vi "运维调试_质控单元.vi"() -> ()   [LabVIEW 2016, in "质控单元.lvlib"]
uses:
  <vilib>/Utility/miscctls.llb/LVPointTypeDef.ctl
  <vilib>/Utility/config.llb/Read Key (I32).vi
  <vilib>/Utility/config.llb/Read Key (Boolean).vi
  <vilib>/Utility/config.llb/Read Key (U32).vi
  <vilib>/Utility/config.llb/Write Key (I32).vi
  <vilib>/Utility/config.llb/Write Key (Boolean).vi
  <vilib>/Utility/config.llb/NI_LVConfig.lvlib
panel:
  in  "标样核查量程选择":enum32{"H", "L", "AUTO"}(ring)=enum."AUTO"
  in  "零点核查量程选择":enum32{"H", "L", "AUTO"}(ring)=enum."AUTO"
  in  "跨度量程选择":enum32{"H", "L", "AUTO"}(ring)=enum."AUTO"
  in  "定时启动":bool
  out "串口/TCP":string
  out "CODCr状态簇":T1
  out "CODMn状态簇":T1
  out "总氮状态簇":T1
  out "总磷状态簇":T1
  out "氨氮状态簇":T1
  out "总氮柱塞泵故障报警":bool
  out "CODCr柱塞泵故障报警":bool
  out "CODMn柱塞泵故障报警":bool
  out "总磷柱塞泵故障报警":bool
  out "氨氮柱塞泵故障报警":bool
  out "总氮传感器故障报警":bool
  out "总氮传感器状态":bool
  out "总氮流程中断报警":bool
  out "总磷通讯":bool
  out "CODCr质控流程中":bool
  out "CODMn质控流程中":bool
  out "总氮质控流程中":bool caption="总磷质控流程中"
  out "总磷质控流程中":bool caption="总氮质控流程中"
  out "氨氮质控流程中":bool
  out "CODCr通讯":bool
  out "CODMn通讯":bool
  out "总氮通讯":bool
  out "氨氮通讯":bool
  out "CODCr传感器状态":bool
  out "CODCr传感器故障报警":bool
  out "CODMn传感器故障报警":bool
  out "总磷传感器故障报警":bool
  out "氨氮传感器故障报警":bool
  out "CODMn传感器状态":bool
  out "总磷传感器状态":bool
  out "氨氮传感器状态":bool
  out "CODCr流程中断报警":bool
  out "总磷流程中断报警":bool
  out "CODMn流程中断报警":bool
  out "氨氮流程中断报警":bool
  in  "总氮模块选择":bool
  in  "释放串口":bool
  in  "打开串口":bool
  in  "柱塞泵调试":bool
  in  "手动调试":bool
  in  "报警清除":bool
  in  "查看":bool
  in  "停止测量":bool
  in  "加标回收":bool
  in  "平行样测试":bool
  in  "CODCr量程选择":enum32{"H", "L", "AUTO"}(ring)
  in  "CODCr选择":bool
  out "CODCr加标回收率":dbl caption="加标回收率" format="%.2f"
  out "CODCr加标体积":dbl caption="加标体积" format="%.3f"
  out "CODCr母液浓度":dbl caption="加标母液浓度" format="%.2f"
  out "CODCr加标水杯定容体积":dbl caption="加标水杯定容体积" format="%.2f"
  out "CODCr加标后水样浓度":dbl caption="加标后水样浓度" format="%.2f"
  out "CODCr加标前水样浓度":dbl caption="加标前水样浓度" format="%.2f"
  out "CODCr检出限":dbl caption="检出限" format="%.2f"
  out "CODCr量程":dbl caption="量程" format="%.2f"
  out "CODCr状态":u16(ring) caption="状态" items=["待机", "润洗", "进样", "进样完成", "柱塞泵加标", "等待取液", "排液"]
  out "质控流程中":bool
  in  "CODMn量程选择":enum32{"H", "L", "AUTO"}(ring)
  in  "总磷量程选择":enum32{"H", "L", "AUTO"}(ring)=enum."AUTO"
  in  "总氮量程选择":enum32{"H", "L", "AUTO"}(ring)=enum."AUTO"
  in  "氨氮量程选择":enum32{"H", "L", "AUTO"}(ring)=enum."AUTO"
  in  "CODMn选择":bool
  in  "总磷模块选择":bool
  in  "氨氮模块":bool
  in  "背隙补偿步数 3":i32 min=0 max=2000
  in  "背隙补偿步数 2":i32 min=0 max=2000
  in  "背隙补偿步数":i32 min=0 max=2000
  out "总氮加标回收率":dbl caption="加标回收率" format="%.2f"
  out "总氮加标体积":dbl caption="加标体积" format="%.3f"
  out "总氮母液浓度":dbl caption="加标母液浓度" format="%.3f"
  out "总氮加标水杯定容体积":dbl caption="加标水杯定容体积" format="%.2f"
  out "总氮加标后水样浓度":dbl caption="加标后水样浓度" format="%.3f"
  out "总氮加标前水样浓度":dbl caption="加标前水样浓度" format="%.3f"
  out "总氮检出限":dbl caption="检出限" format="%.3f"
  out "总氮量程":dbl caption="量程" format="%.2f"
  out "总氮状态":u16(ring) caption="状态" items=["待机", "润洗", "进样", "进样完成", "柱塞泵加标", "等待取液", "排液"]
  in  "返回":bool
  out "COD平行样测完标志":bool
  out "氨氮总磷平行样测完标志":bool
  out "COD加标回收率":dbl caption="加标回收率" format="%.2f"
  out "COD加标体积":dbl caption="加标体积" format="%.3f"
  out "COD母液浓度":dbl caption="加标母液浓度" format="%.2f"
  out "COD加标水杯定容体积":dbl caption="加标水杯定容体积" format="%.2f"
  out "COD加标后水样浓度":dbl caption="加标后水样浓度" format="%.2f"
  out "COD加标前水样浓度":dbl caption="加标前水样浓度" format="%.2f"
  out "COD检出限":dbl caption="检出限" format="%.2f"
  out "COD量程":dbl caption="量程" format="%.2f"
  out "CODMn状态":u16(ring) caption="状态" items=["待机", "润洗", "进样", "进样完成", "柱塞泵加标", "等待取液", "排液"]
  out "总磷加标回收率":dbl caption="加标回收率" format="%.2f"
  out "总磷加标体积":dbl caption="加标体积" format="%.3f"
  out "总磷母液浓度":dbl caption="加标母液浓度" format="%.3f"
  out "总磷加标水杯定容体积":dbl caption="加标水杯定容体积" format="%.2f"
  out "总磷加标后水样浓度":dbl caption="加标后水样浓度" format="%.3f"
  out "总磷加标前水样浓度":dbl caption="加标前水样浓度" format="%.3f"
  out "总磷检出限":dbl caption="检出限" format="%.3f"
  out "总磷量程":dbl caption="量程" format="%.2f"
  out "总磷状态":u16(ring) caption="状态" items=["待机", "润洗", "进样", "进样完成", "柱塞泵加标", "等待取液", "排液"]
  out "氨氮加标回收率":dbl caption="加标回收率" format="%.2f"
  out "氨氮加标体积":dbl caption="加标体积" format="%.3f"
  out "氨氮母液浓度":dbl caption="加标母液浓度" format="%.3f"
  out "氨氮加标水杯定容体积":dbl caption="加标水杯定容体积" format="%.2f"
  out "氨氮加标后水样浓度":dbl caption="加标后水样浓度" format="%.3f"
  out "氨氮加标前水样浓度":dbl caption="加标前水样浓度" format="%.3f"
  out "氨氮检出限":dbl caption="检出限" format="%.3f"
  out "氨氮量程":dbl caption="量程" format="%.2f"
  out "氨氮状态":u16(ring) caption="状态" items=["待机", "润洗", "进样", "进样完成", "柱塞泵加标", "等待取液", "排液"]
  # "氨氮质控参数"
  # "状态显示区"
  # "参数配置区"
  # "2000步等于1mL\n100步等于0.05mL\n20步等于0.01mL\n2步等于0.001mL\n（初始默认100步）"
  # "柱塞泵调试区"
  # "CODCr质控参数"
  # "%"
  # "mL"
  # "mg/L"
  # "mL"
  # "mg/L"
  # "mg/L"
  # "mg/L"
  # "mg/L"
  # "总氮质控参数"
  # "%"
  # "mL"
  # "mg/L"
  # "mL"
  # "mg/L"
  # "mg/L"
  # "mg/L"
  # "mg/L"
  # "CODMn质控参数"
  # "%"
  # "mL"
  # "mg/L"
  # "mL"
  # "mg/L"
  # "mg/L"
  # "mg/L"
  # "mg/L"
  # "总磷质控参数"
  # "%"
  # "mL"
  # "mg/L"
  # "mL"
  # "mg/L"
  # "mg/L"
  # "mg/L"
  # "mg/L"
  # "%"
  # "mL"
  # "mg/L"
  # "mL"
  # "mg/L"
  # "mg/L"
  # "mg/L"
  # "mg/L"
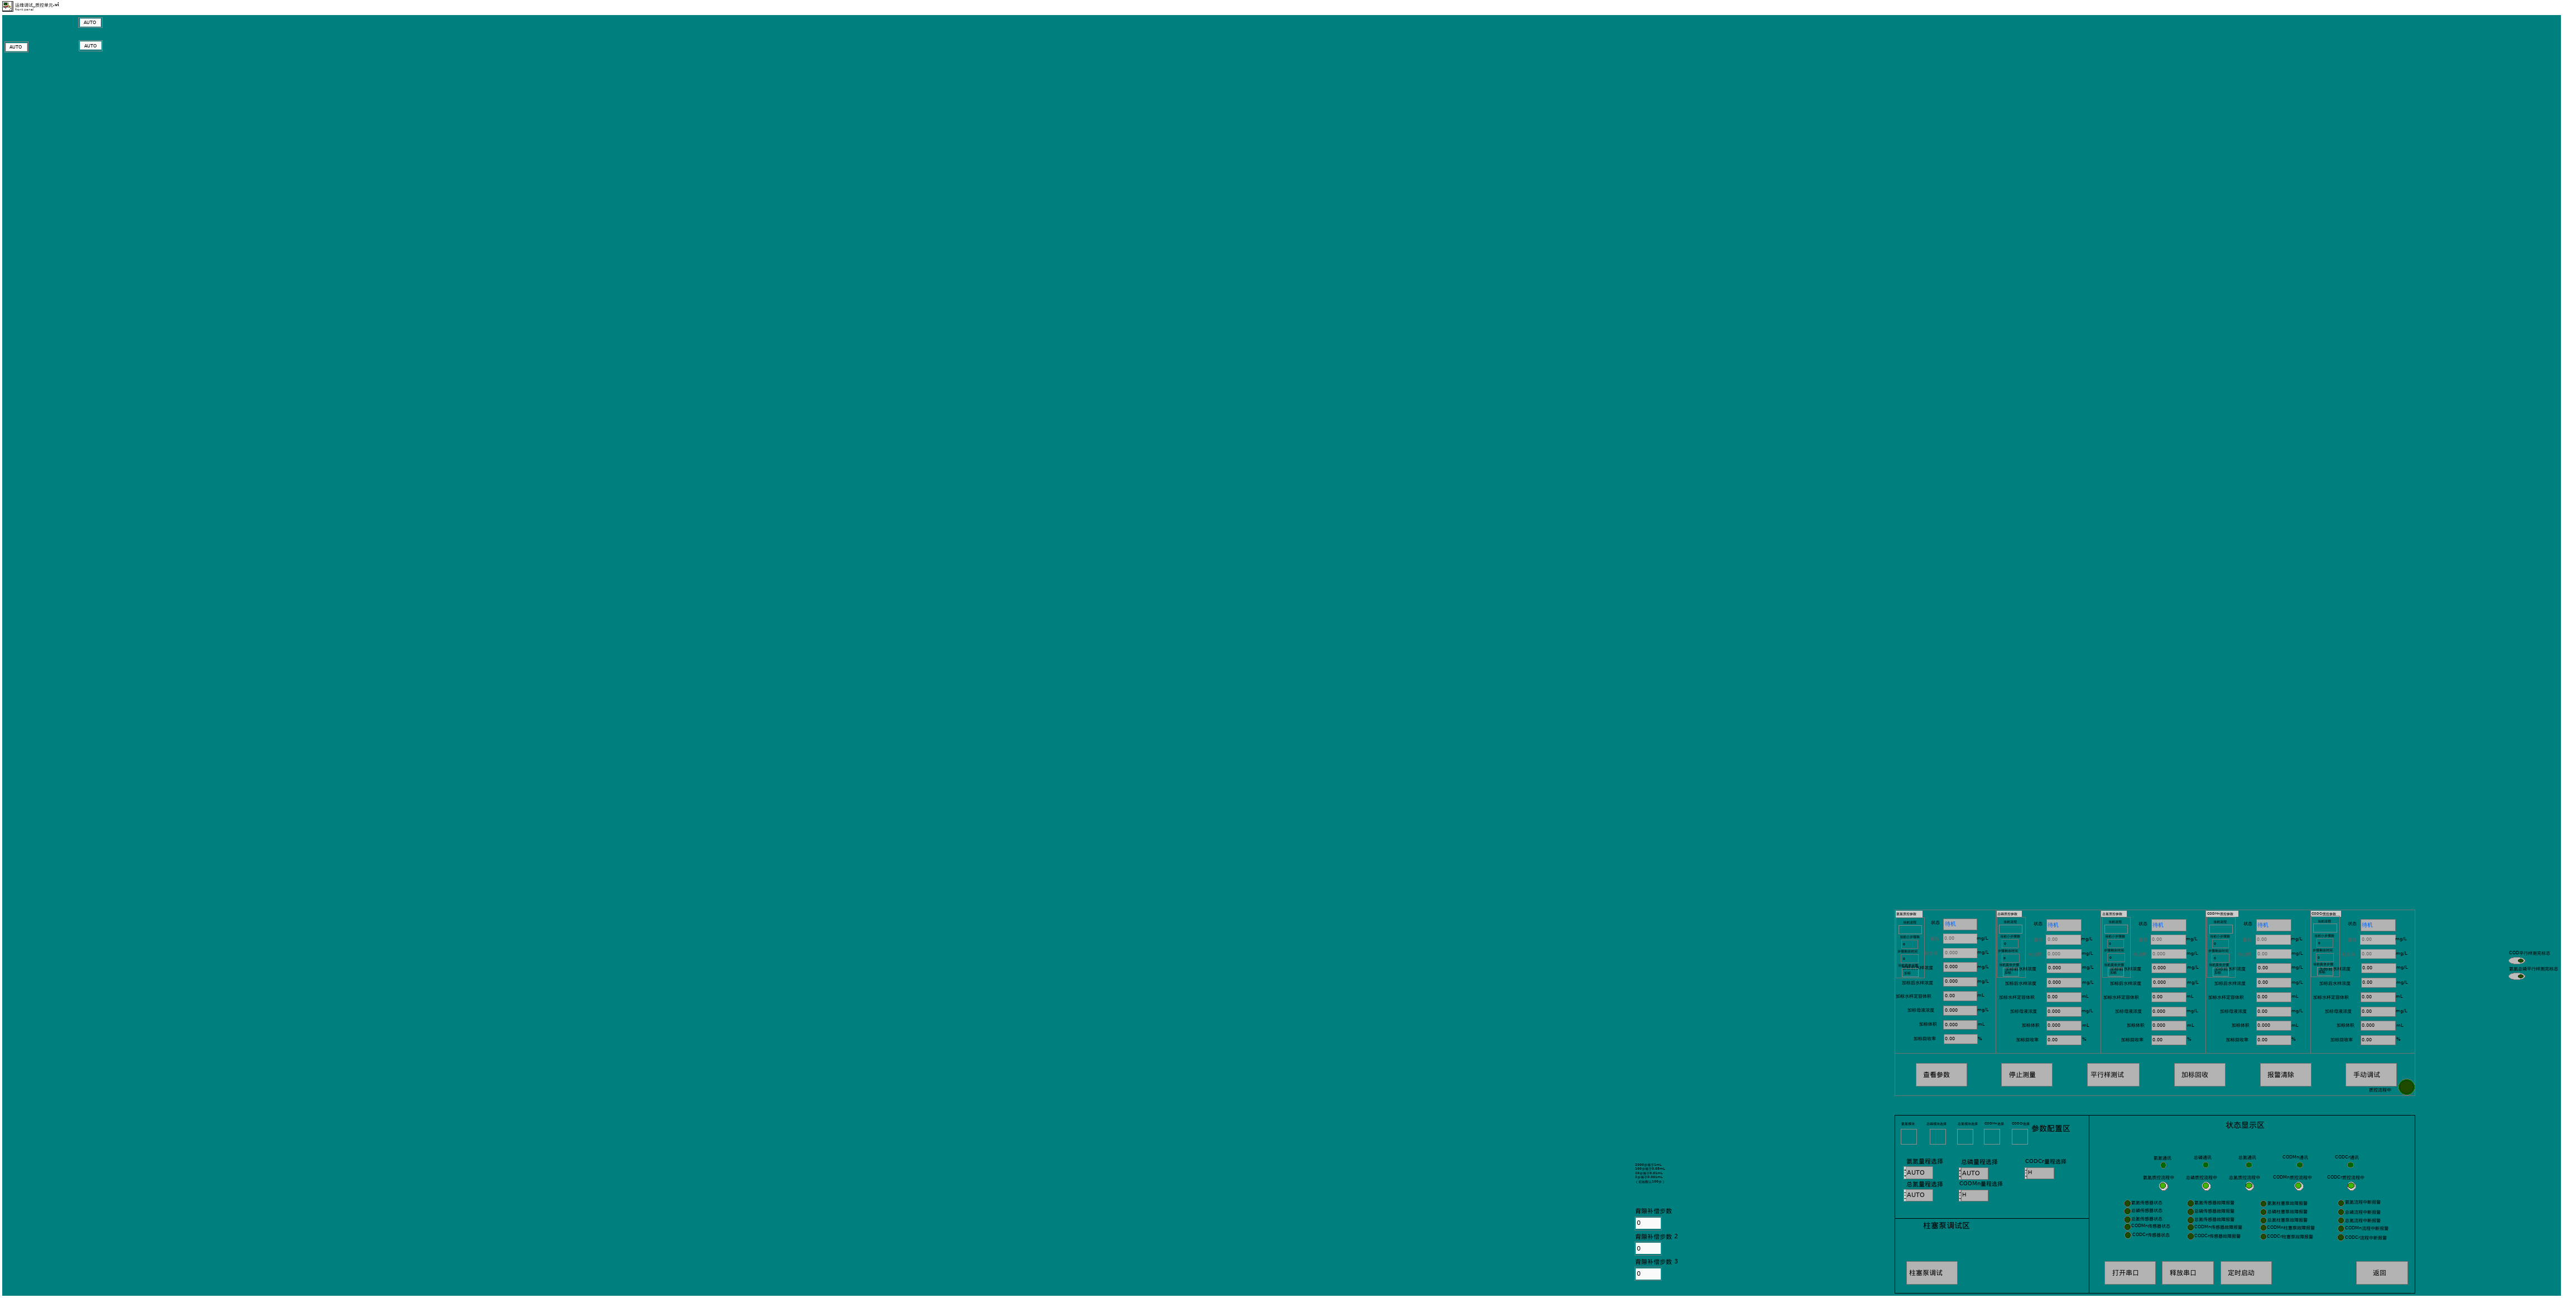
[diagram p1: front panel]
types:
  T1 = cluster{"步骤剩余时间":u16, "当前具体步骤":enum16{"加标", "进样", "排液", "搅拌", "定量"}, " 当前流程":enum16{"", "水样流程", "加标流程", "排液流程"}, "当前小步骤数":i8}
  T2 = typedef "LVPointTypeDef.ctl" = cluster{"Horizontal":i16, "Vertical":i16}
  T3 = typedef "NI_LVConfig.lvlib/Config Data RefNum.ctl" = refnum<k1>
  T4 = cluster{"量程":dbl, "检出限":dbl, "加标前水样浓度":dbl, "加标后水样浓度":dbl, "加标水杯定容体积":dbl, "加标母液浓度":dbl, "加标体积":dbl, "加标回收率":dbl}
  T5 = enum8{"Enabled", "Disabled", "Disabled and Grayed Out"}
  T6 = cluster{"周期设置类型":enum16{"定点启动", "间隔启动"}, "定时功能启用":bool, "定时间隔":dbl, "24H周期设置":bool[], "模块选择":cluster{"氨氮":bool, "总磷":bool, "总氮":bool, "CODMn":bool, "CODCr":bool}}
  T7 = typedef "LVDateTimeRec.ctl" = cluster{"秒数的小数部分":dbl, "秒":i32, "分":i32, "时":i32, "日":i32, "月":i32, "年":i32, "天数（周）":i32, "天数（年）":i32, "DST":i32}
  T8 = cluster{"氨氮":bool, "总磷":bool, "总氮":bool, "CODMn":bool, "CODCr":bool}
  T9 = cluster{"是否启用仪器":bool, "CODMn":cluster{"启动测量模式":cluster{"测量模式":enum16{"水样测量", "标样核查", "加标回收", "平行样", "校零", "校标"}}, "确定按钮":bool}, "启动模块":cluster{"氨氮":bool, "总磷":bool, "总氮":bool, "CODMn":bool, "CODCr":bool}, "常规启动":bool, "直接启动":bool}
  T10 = cluster{"参数启用":cluster{"CODMn":bool, "总磷":bool, "总氮":bool, "氨氮":bool, "CODcr":bool}, "采配水是否启动":bool}
  T11 = cluster{"命令":string, cluster{"starting address":u16, "holding register value":u16}}
  T12 = enum32{"Bad", "Idle", "Run top level", "Running"}
  T13 = cluster{"CODMn":bool, "总磷":bool, "总氮":bool, "氨氮":bool, "CODCr":bool}
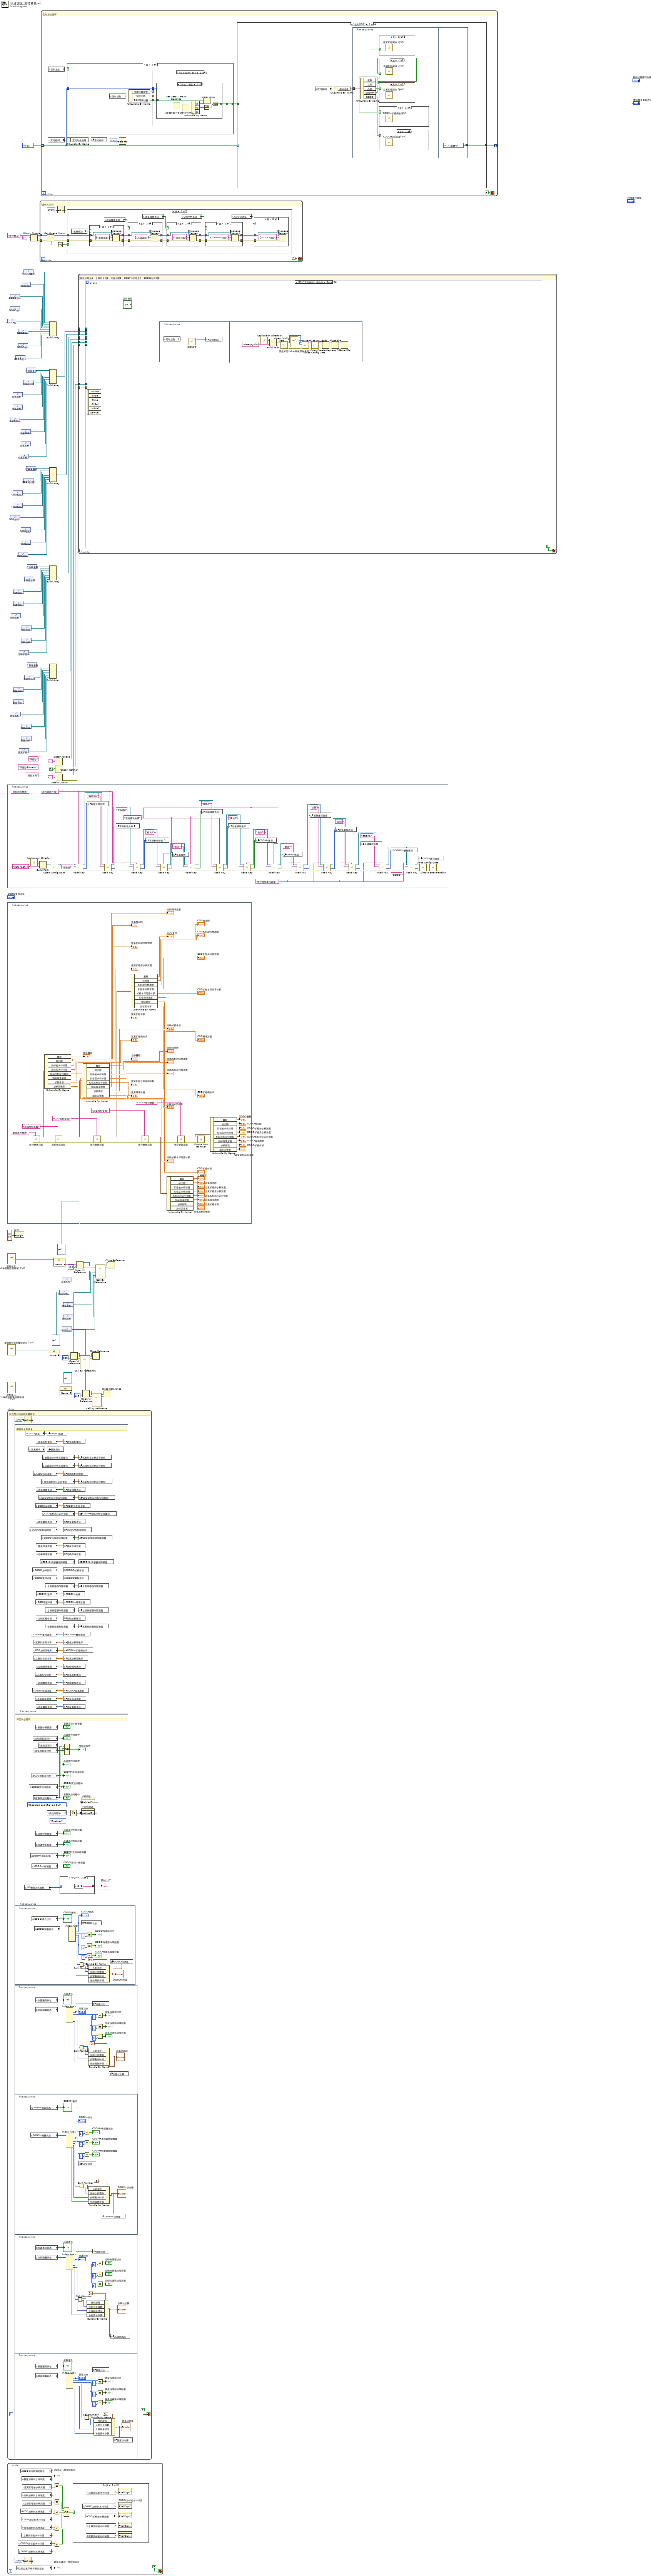
[diagram p0: block diagram]
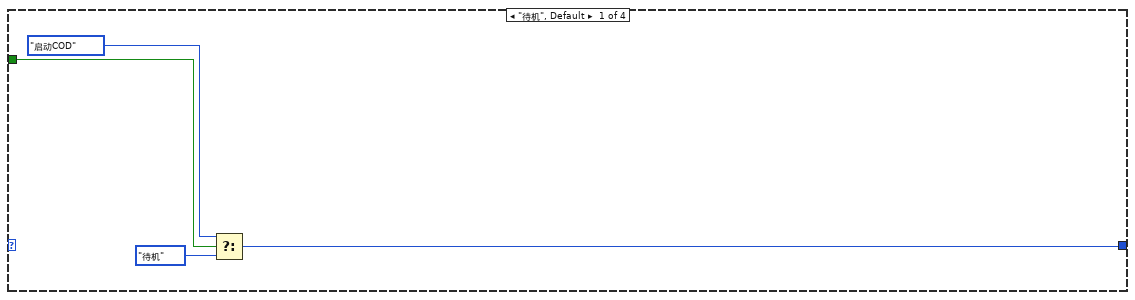
[diagram p2: hidden frame]
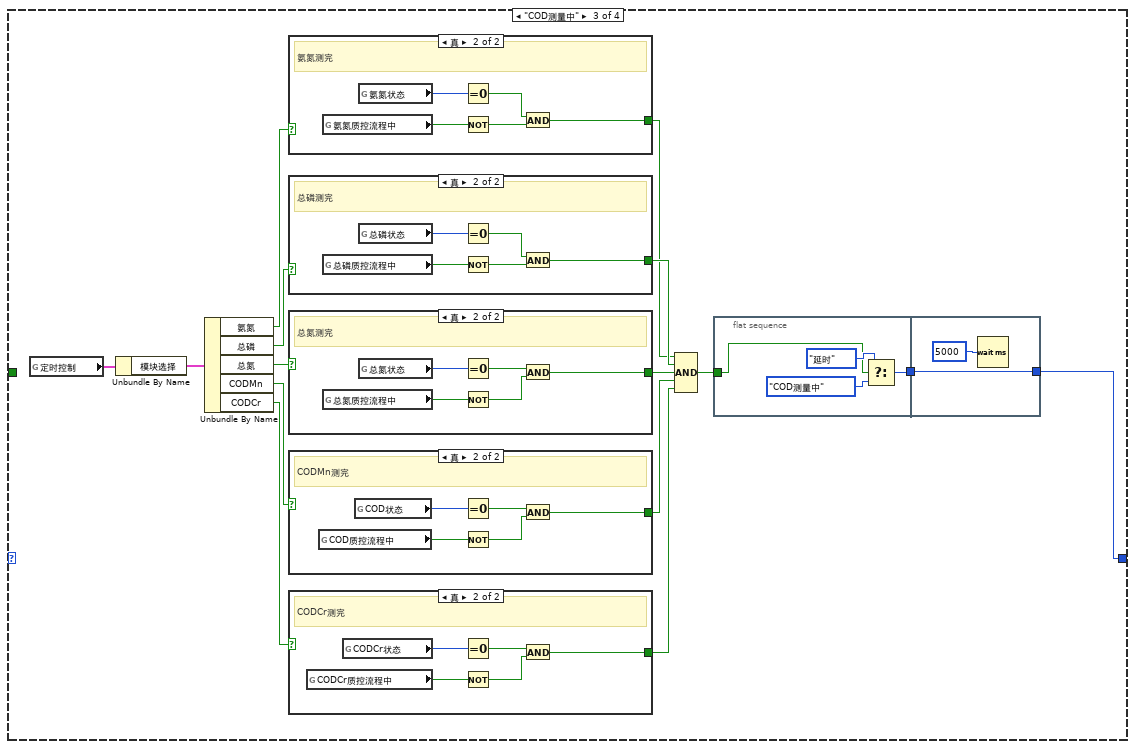
[diagram p8: hidden frame]
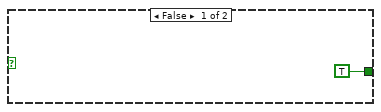
[diagram p9: hidden frame]
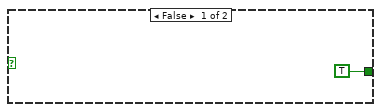
[diagram p10: hidden frame]
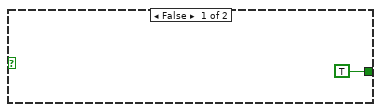
[diagram p11: hidden frame]
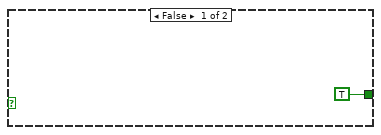
[diagram p12: hidden frame]
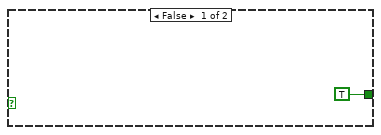
[diagram p13: hidden frame]
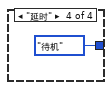
[diagram p14: hidden frame]
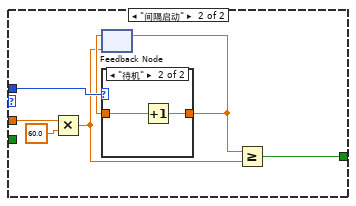
[diagram p17: hidden frame]
diagram:
  n1 = control-ref of="CODCr加标水杯定容体积"() -> (w43:refnum<vi>)
  n2 = flat-sequence {
    frame #0 {
      w111 = "质控模块量程选择" ("section")
      w92 = "质控模块选择" ("section")
      (unwired) "质控线性参数" ("section")
      w145 = "质控背隙补偿" ("section")
      n3 = call <vilib>:"Application Directory.vi"() -> ("Application Directory"=w151:path)
      n4 = Build Path(base path=w151, name or relative path="data\\Set.ini" ("名称或相对路径")) -> (appended path=w149:path)
      n5 = call <vilib>:"Open Config Data.vi"("configuration file path"=w149) -> ("error out"=w147:errorcluster, "refnum"=w148:T3)  [unwired: 8 in, 1 out]
      n6 = call-poly <vilib>:"Read Key.vi"("section"=w145, "error in (no error)"=w147, "key"="背隙值1", "refnum"=w148) -> ("error out"=w142:errorcluster, "value"=w137:i32, "refnum out"=w144:T3)  [unwired: 4 in, 1 out]
      n7 = local write "背隙补偿步数"(w137) -> ()
      n8 = call-poly <vilib>:"Read Key.vi"("section"=w145, "error in (no error)"=w142, "key"="背隙值2", "refnum"=w144) -> ("error out"=w140:errorcluster, "value"=w138:i32, "refnum out"=w141:T3)  [unwired: 4 in, 1 out]
      n9 = local write "背隙补偿步数 2"(w138) -> ()
      n10 = call-poly <vilib>:"Read Key.vi"("section"=w145, "error in (no error)"=w140, "key"="背隙值3", "refnum"=w141) -> ("error out"=w99:errorcluster, "value"=w136:i32, "refnum out"=w100:T3)  [unwired: 4 in, 1 out]
      n11 = local write "背隙补偿步数 3"(w136) -> ()
      n12 = call-poly <vilib>:"Read Key.vi"("section"=w92, "error in (no error)"=w99, "key"="模块1" ("section"), "refnum"=w100) -> ("error out"=w134:errorcluster, "value"=w128:bool, "refnum out"=w135:T3)  [unwired: 4 in, 1 out]
      n13 = local write "氨氮模块"(w128) -> ()
      n14 = call-poly <vilib>:"Read Key.vi"("section"=w92, "error in (no error)"=w134, "key"="模块2" ("section"), "refnum"=w135) -> ("error out"=w96:errorcluster, "value"=w129:bool, "refnum out"=w97:T3)  [unwired: 4 in, 1 out]
      n15 = local write "总磷模块选择"(w129) -> ()
      n16 = call-poly <vilib>:"Read Key.vi"("section"=w92, "error in (no error)"=w96, "key"="模块3" ("section"), "refnum"=w97) -> ("error out"=w94:errorcluster, "value"=w93:bool, "refnum out"=w95:T3)  [unwired: 4 in, 1 out]
      n17 = local write "总氮模块选择"(w93) -> ()
      n18 = call-poly <vilib>:"Read Key.vi"("section"=w92, "error in (no error)"=w94, "key"="模块4" ("section"), "refnum"=w95) -> ("error out"=w105:errorcluster, "value"=w130:bool, "refnum out"=w106:T3)  [unwired: 4 in, 1 out]
      n19 = local write "CODMn选择"(w130) -> ()
      n20 = call-poly <vilib>:"Read Key.vi"("section"=w92, "error in (no error)"=w105, "key"="模块5", "refnum"=w106) -> ("error out"=w102:errorcluster, "value"=w101:bool, "refnum out"=w103:T3)  [unwired: 4 in, 1 out]
      n21 = local write "CODCr选择"(w101) -> ()
      n22 = call-poly <vilib>:"Read Key.vi"("section"=w111, "error in (no error)"=w102, "key"="氨氮" ("section"), "refnum"=w103) -> ("error out"=w126:errorcluster, "value"=w117:u32, "refnum out"=w127:T3)  [unwired: 4 in, 1 out]
      n23 = local write "氨氮量程选择"(w117) -> ()
      n24 = call-poly <vilib>:"Read Key.vi"("section"=w111, "error in (no error)"=w126, "key"="总氮" ("section"), "refnum"=w127) -> ("error out"=w124:errorcluster, "value"=w116:u32, "refnum out"=w125:T3)  [unwired: 4 in, 1 out]
      n25 = local write "总氮量程选择"(w116) -> ()
      n26 = call-poly <vilib>:"Read Key.vi"("section"=w111, "error in (no error)"=w124, "key"="总磷" ("section"), "refnum"=w125) -> ("error out"=w122:errorcluster, "value"=w115:u32, "refnum out"=w123:T3)  [unwired: 4 in, 1 out]
      n27 = local write "总磷量程选择"(w115) -> ()
      n28 = call-poly <vilib>:"Read Key.vi"("section"=w111, "error in (no error)"=w122, "key"="CODMn" ("section"), "refnum"=w123) -> ("error out"=w112:errorcluster, "value"=w114:u32, "refnum out"=w113:T3)  [unwired: 4 in, 1 out]
      n29 = local write "CODMn量程选择"(w114) -> ()
      n30 = call-poly <vilib>:"Read Key.vi"("section"=w111, "error in (no error)"=w112, "key"="CODCr" ("section"), "refnum"=w113) -> ("error out"=w108:errorcluster, "value"=w109:u32, "refnum out"=w107:T3)  [unwired: 4 in, 1 out]
      n31 = local write "CODCr量程选择"(w109) -> ()
      n32 = call <vilib>:"Close Config Data.vi"("error in (no error)"=w108, "refnum"=w107) -> ("error out"=w91:errorcluster)  [unwired: 8 in, 1 out]
      n33 = call <vilib>:"Simple Error Handler.vi"("error in (no error)"=w91) -> ()  [unwired: 4 in, 5 out]
    }
  }
  n34 = flat-sequence {
    frame #0 {
      n35 = call "质控参数读取.vi"("section"="氨氮质控参数") -> ("error out"=w186:errorcluster, "参数"=w205:T4)  [unwired: 9 in]
      n36 = Unbundle By Name(w205) -> ("量程"=→"氨氮量程":dbl, "检出限"=→"氨氮检出限":dbl, "加标前水样浓度"=→"氨氮加标前水样浓度":dbl, "加标后水样浓度"=→"氨氮加标后水样浓度":dbl, "加标水杯定容体积"=→"氨氮加标水杯定容体积":dbl, "加标母液浓度"=→"氨氮母液浓度":dbl, "加标体积"=→"氨氮加标体积":dbl, "加标回收率"=→"氨氮加标回收率":dbl)
      n37 = call "质控参数读取.vi"("section"="总磷质控参数", "error in (no error)"=w186) -> ("error out"=w183:errorcluster, "参数"=w195:T4)  [unwired: 8 in]
      n38 = Unbundle By Name(w195) -> ("量程"=→"总磷量程":dbl, "检出限"=→"总磷检出限":dbl, "加标前水样浓度"=→"总磷加标前水样浓度":dbl, "加标后水样浓度"=→"总磷加标后水样浓度":dbl, "加标水杯定容体积"=→"总磷加标水杯定容体积":dbl, "加标母液浓度"=→"总磷母液浓度":dbl, "加标体积"=→"总磷加标体积":dbl, "加标回收率"=→"总磷加标回收率":dbl)
      n39 = call "质控参数读取.vi"("section"="COD质控参数", "error in (no error)"=w183) -> ("error out"=w173:errorcluster, "参数"=w185:T4)  [unwired: 8 in]
      n40 = Unbundle By Name(w185) -> ("量程"=→"COD量程":dbl, "检出限"=→"COD检出限":dbl, "加标前水样浓度"=→"COD加标前水样浓度":dbl, "加标后水样浓度"=→"COD加标后水样浓度":dbl, "加标水杯定容体积"=→"COD加标水杯定容体积":dbl, "加标母液浓度"=→"COD母液浓度":dbl, "加标体积"=→"COD加标体积":dbl, "加标回收率"=→"COD加标回收率":dbl)
      n41 = call "质控参数读取.vi"("section"="总氮质控参数", "error in (no error)"=w173) -> ("error out"=w161:errorcluster, "参数"=w172:T4)  [unwired: 8 in]
      n42 = Unbundle By Name(w172) -> ("量程"=→"总氮量程":dbl, "检出限"=→"总氮检出限":dbl, "加标前水样浓度"=→"总氮加标前水样浓度":dbl, "加标后水样浓度"=→"总氮加标后水样浓度":dbl, "加标水杯定容体积"=→"总氮加标水杯定容体积":dbl, "加标母液浓度"=→"总氮母液浓度":dbl, "加标体积"=→"总氮加标体积":dbl, "加标回收率"=→"总氮加标回收率":dbl)
      n43 = call "质控参数读取.vi"("section"="CODCr质控参数", "error in (no error)"=w161) -> ("error out"=w152:errorcluster, "参数"=w162:T4)  [unwired: 8 in]
      n44 = call <vilib>:"Simple Error Handler.vi"("error in (no error)"=w152) -> ()  [unwired: 4 in, 5 out]
      n45 = Unbundle By Name(w162) -> ("量程"=→"CODCr量程":dbl, "检出限"=→"CODCr检出限":dbl, "加标前水样浓度"=→"CODCr加标前水样浓度":dbl, "加标后水样浓度"=→"CODCr加标后水样浓度":dbl, "加标水杯定容体积"=→"CODCr加标水杯定容体积":dbl, "加标母液浓度"=→"CODCr母液浓度":dbl, "加标体积"=→"CODCr加标体积":dbl, "加标回收率"=→"CODCr加标回收率":dbl)
    }
  }
  n46 = vi-ref "质控单元.lvlib:质控数据存储(子VI).vi"() -> (w18:refnum<vi>)
  n47 = vi-ref "通信并与其他模块交互 (子VI).vi"() -> (w31:refnum<vi>)
  n48 = vi-ref "质控单元.lvlib:质控报警信息存储 (子VI).vi"() -> (w26:refnum<vi>)
  n49 = while {
    stop <- FALSE stop-if-true
    # "状态显示和全局变量赋值"
    n50 = flat-sequence {
      frame #0 {
        # "赋值给全局变量"
        n51 = local read "CODCr选择"() -> (w346:bool)
        n52 = local read "氨氮模块"() -> (w345:bool)
        n53 = local read "CODCr加标回收率"() -> (w328:dbl)
        n54 = local read "CODMn量程选择"() -> (w352:enum32{"H", "L", "AUTO"})
        n55 = local read "CODCr加标体积"() -> (w339:dbl)
        n56 = local read "CODCr量程选择"() -> (w353:enum32{"H", "L", "AUTO"})
        n57 = local read "CODCr母液浓度"() -> (w329:dbl)
        n58 = local read "COD加标回收率"() -> (w327:dbl)
        n59 = local read "总磷加标回收率"() -> (w325:dbl)
        n60 = local read "氨氮加标回收率"() -> (w324:dbl)
        n61 = local read "总氮加标回收率"() -> (w326:dbl)
        n62 = local read "总氮加标体积"() -> (w341:dbl)
        n63 = local read "总氮母液浓度"() -> (w331:dbl)
        n64 = local read "COD加标体积"() -> (w340:dbl)
        n65 = local read "COD母液浓度"() -> (w330:dbl)
        n66 = local read "氨氮加标体积"() -> (w343:dbl)
        n67 = local read "总氮模块选择"() -> (w348:bool)
        n68 = local read "氨氮量程选择"() -> (w351:enum32{"H", "L", "AUTO"})
        n69 = local read "氨氮母液浓度"() -> (w333:dbl)
        n70 = local read "总磷母液浓度"() -> (w332:dbl)
        n71 = local read "总磷加标体积"() -> (w342:dbl)
        n72 = local read "总磷模块选择"() -> (w344:bool)
        n73 = local read "总磷量程选择"() -> (w349:enum32{"H", "L", "AUTO"})
        n74 = local read "总氮量程选择"() -> (w350:enum32{"H", "L", "AUTO"})
        n75 = local read "CODMn选择"() -> (w347:bool)
        n76 = local read "CODCr加标水杯定容体积"() -> (w338:dbl)
        n77 = local read "CODMn传感器故障报警"() -> (w320:bool)
        n78 = local read "总氮加标水杯定容体积"() -> (w336:dbl)
        n79 = local read "CODCr传感器故障报警"() -> (w319:bool)
        n80 = local read "COD加标水杯定容体积"() -> (w337:dbl)
        n81 = local read "氨氮加标水杯定容体积"() -> (w334:dbl)
        n82 = local read "总磷加标水杯定容体积"() -> (w335:dbl)
        n83 = local read "总氮传感器故障报警"() -> (w321:bool)
        n84 = local read "总磷传感器故障报警"() -> (w322:bool)
        n85 = local read "氨氮传感器故障报警"() -> (w323:bool)
        n86 = global write "断电保存全局.vi" "CODCr选择"(w346) -> ()
        n87 = global write "断电保存全局.vi" "氨氮模块"(w345) -> ()
        n88 = global write "加标回收状态全局变量.vi" "氨氮加标体积"(w343) -> ()
        n89 = global write "加标回收状态全局变量.vi" "总磷加标回收率"(w325) -> ()
        n90 = global write "断电保存全局.vi" "总氮模块选择"(w348) -> ()
        n91 = global write "加标回收状态全局变量.vi" "CODMn加标体积"(w340) -> ()
        n92 = global write "断电保存全局.vi" "氨氮量程选择"(w351) -> ()
        n93 = global write "加标回收状态全局变量.vi" "CODCr加标回收率"(w328) -> ()
        n94 = global write "加标回收状态全局变量.vi" "氨氮母液浓度"(w333) -> ()
        n95 = global write "加标回收状态全局变量.vi" "总磷母液浓度"(w332) -> ()
        n96 = global write "加标回收状态全局变量.vi" "CODCr加标体积"(w339) -> ()
        n97 = global write "断电保存全局.vi" "CODCr量程选择"(w353) -> ()
        n98 = global write "断电保存全局.vi" "CODMn选择"(w347) -> ()
        n99 = global write "加标回收状态全局变量.vi" "CODMn母液浓度"(w330) -> ()
        n100 = global write "加标回收状态全局变量.vi" "总磷加标体积"(w342) -> ()
        n101 = global write "断电保存全局.vi" "CODMn量程选择"(w352) -> ()
        n102 = global write "加标回收状态全局变量.vi" "氨氮加标回收率"(w324) -> ()
        n103 = global write "加标回收状态全局变量.vi" "CODMn加标回收率"(w327) -> ()
        n104 = global write "加标回收状态全局变量.vi" "总氮加标回收率"(w326) -> ()
        n105 = global write "断电保存全局.vi" "总磷模块选择"(w344) -> ()
        n106 = global write "加标回收状态全局变量.vi" "总氮加标体积"(w341) -> ()
        n107 = global write "断电保存全局.vi" "总磷量程选择"(w349) -> ()
        n108 = global write "加标回收状态全局变量.vi" "CODCr母液浓度"(w329) -> ()
        n109 = global write "加标回收状态全局变量.vi" "总氮母液浓度"(w331) -> ()
        n110 = global write "断电保存全局.vi" "总氮量程选择"(w350) -> ()
        n111 = global write "加标回收状态全局变量.vi" "氨氮加标水杯定容体积"(w334) -> ()
        n112 = global write "加标回收状态全局变量.vi" "总磷加标水杯定容体积"(w335) -> ()
        n113 = global write "加标回收状态全局变量.vi" "总氮加标水杯定容体积"(w336) -> ()
        n114 = global write "加标回收状态全局变量.vi" "CODCr加标水杯定容体积"(w338) -> ()
        n115 = global write "加标回收状态全局变量.vi" "CODMn加标水杯定容体积"(w337) -> ()
        n116 = global write "质控中断报警全局.vi" "CODCr传感器故障报警"(w319) -> ()
        n117 = global write "质控中断报警全局.vi" "CODMn传感器故障报警"(w320) -> ()
        n118 = global write "质控中断报警全局.vi" "总氮传感器故障报警"(w321) -> ()
        n119 = global write "质控中断报警全局.vi" "总磷传感器故障报警"(w322) -> ()
        n120 = global write "质控中断报警全局.vi" "氨氮传感器故障报警"(w323) -> ()
      }
    }
    n121 = flat-sequence {
      frame #0 {
        # "界面状态显示"
        n122 = global read "断电保存全局.vi" "MB通信方式选择"() -> (w300:enum16{"串口", "TCP"})
        n123 = global read "质控测完标志全局 1.vi" "CODCr质控流程中"() -> (w307:bool)
        "CODCr质控流程中" <- w307
        n124 = global read "质控中断报警全局.vi" "CODMn中断报警"() -> (→"CODMn流程中断报警":bool)
        n125 = global read "质控测完标志全局 1.vi" "COD质控流程中"() -> (w306:bool)
        "CODMn质控流程中" <- w306
        n126 = global read "质控中断报警全局.vi" "CODCr中断报警"() -> (→"CODCr流程中断报警":bool)
        n127 = global read "质控测完标志全局 1.vi" "总磷质控流程中"() -> (w305:bool)
        "总磷质控流程中" <- w305
        n128 = global read "质控测完标志全局 1.vi" "总氮质控流程中"() -> (w308:bool)
        "总氮质控流程中" <- w308
        n129 = global read "质控测完标志全局 1.vi" "氨氮质控流程中"() -> (w304:bool)
        "氨氮质控流程中" <- w304
        n130 = global read "质控中断报警全局.vi" "氨氮中断报警"() -> (→"氨氮流程中断报警":bool)
        n131 = global read "质控中断报警全局.vi" "总氮中断报警"() -> (→"总氮流程中断报警":bool)
        n132 = global read "质控中断报警全局.vi" "总磷中断报警"() -> (→"总磷流程中断报警":bool)
        n133 = global read "质控测完标志全局 1.vi" "质控流程中"() -> (w302:bool)
        n134 = global read "质控测完标志全局 1.vi" "质控流程中"() -> (w312:bool)
        n135 = case shown="\"TCP\"" w300 {
          tunnel: [w317 w318] -> w299
          frame "串口", Default {
            n136 = global read "断电保存全局.vi" "VISA Resource"() -> (w317:refnum<visa-resource-name>)
          }
          frame "TCP" {
            n137 = global read "断电保存全局.vi" "IP"() -> (w318:string)
          }
        }
        "串口/TCP" <- w299
        n138 = Compound Arithmetic op=OR ("复合运算")(w302, w304, w305, w308, w306, w307) -> (→"质控流程中":bool)
        n139 = Select(t=T5."Disabled and Grayed Out" ("禁用"), s=w312, f=T5."Enabled") -> (s? t:f=w301:T5)
        n140 = property on="平行样测试" class="Bool"("DisabledEnum"=w301) -> ()  [unwired: 2 in, 2 out]
        n141 = property on="加标回收" class="Bool"("DisabledEnum"=w301) -> ()  [unwired: 2 in, 2 out]
      }
    }
    n142 = flat-sequence {
      frame #0 {
        n143 = global read "质控内部交互全局.vi" "CODCr通讯状态"() -> (→"CODCr通讯":bool)
        n144 = global read "质控内部交互全局.vi" "CODCr测量状态"() -> (w243:u16[])
        n145 = Index Array(array=w243) -> (element #1=w244:u16, element #2=w239:u16, element #3=w235:u16, element #4=w233:u16, element #5=w230:u16, element #6=w229:u16)  [unwired: 6 in]
        "CODCr状态" <- w244
        n146 = Split Number(x=w233) -> (hi(x)=w232:u8, lo(x)=w231:u8)
        n147 = global write "加标回收状态全局变量.vi" "CODCr状态"(w244) -> ()
        n148 = Equal?(x=w239, y=u16 1) -> (x = y?=→"CODCr传感器状态":bool)
        n149 = Equal?(x=w235, y=u16 1) -> (x = y?=→"CODCr传感器故障报警":bool)
        n150 = Equal?(x=w235, y=u16 2) -> (x = y?=→"CODCr柱塞泵故障报警":bool)
        n151 = Bundle By Name(cluster=T1 {"步骤剩余时间"=0, "当前具体步骤"=enum."加标", " 当前流程"=enum."", "当前小步骤数"=0} ("氨氮状态簇"), "当前流程"=w232, "当前小步骤数"=w231, "步骤剩余时间"=w230, "当前具体步骤"=w229) -> (w227:T1)
        "CODCr状态簇" <- w227
        n152 = global write "加标回收状态全局变量.vi" "CODCr状态簇"(w227) -> ()
      }
    }
    n153 = flat-sequence {
      frame #0 {
        n154 = global read "质控内部交互全局.vi" "总氮通讯状态"() -> (→"总氮通讯":bool)
        n155 = global read "质控内部交互全局.vi" "总氮测量状态"() -> (w223:u16[])
        n156 = Index Array(array=w223) -> (element #1=w222:u16, element #2=w225:u16, element #3=w217:u16, element #4=w213:u16, element #5=w211:u16, element #6=w212:u16)  [unwired: 6 in]
        "总氮状态" <- w222
        n157 = Split Number(x=w213) -> (hi(x)=w215:u8, lo(x)=w214:u8)
        n158 = Bundle By Name(cluster=T1 {"步骤剩余时间"=0, "当前具体步骤"=enum."加标", " 当前流程"=enum."", "当前小步骤数"=0} ("氨氮状态簇"), "当前流程"=w215, "当前小步骤数"=w214, "步骤剩余时间"=w211, "当前具体步骤"=w212) -> (w209:T1)
        "总氮状态簇" <- w209
        n159 = global write "加标回收状态全局变量.vi" "总氮状态"(w222) -> ()
        n160 = Equal?(x=w225, y=u16 1) -> (x = y?=→"总氮传感器状态":bool)
        n161 = Equal?(x=w217, y=u16 1) -> (x = y?=→"总氮传感器故障报警":bool)
        n162 = Equal?(x=w217, y=u16 2) -> (x = y?=→"总氮柱塞泵故障报警":bool)
        n163 = global write "加标回收状态全局变量.vi" "总氮状态簇"(w209) -> ()
      }
    }
    n164 = flat-sequence {
      frame #0 {
        n165 = global read "质控内部交互全局.vi" "CODMn通讯状态"() -> (→"CODMn通讯":bool)
        n166 = global read "质控内部交互全局.vi" "CODMn测量状态"() -> (w259:u16[])
        n167 = Index Array(array=w259) -> (element #1=w262:u16, element #2=w260:u16, element #3=w253:u16, element #4=w249:u16, element #5=w247:u16, element #6=w248:u16)  [unwired: 6 in]
        "CODMn状态" <- w262
        n168 = Split Number(x=w249) -> (hi(x)=w251:u8, lo(x)=w250:u8)
        n169 = global write "加标回收状态全局变量.vi" "COD状态"(w262) -> ()
        n170 = Equal?(x=w260, y=u16 1) -> (x = y?=→"CODMn传感器状态":bool)
        n171 = Equal?(x=w253, y=u16 1) -> (x = y?=→"CODMn传感器故障报警":bool)
        n172 = Equal?(x=w253, y=u16 2) -> (x = y?=→"CODMn柱塞泵故障报警":bool)
        n173 = Bundle By Name(cluster=T1 {"步骤剩余时间"=0, "当前具体步骤"=enum."加标", " 当前流程"=enum."", "当前小步骤数"=0} ("氨氮状态簇"), "当前流程"=w251, "当前小步骤数"=w250, "步骤剩余时间"=w247, "当前具体步骤"=w248) -> (w245:T1)
        "CODMn状态簇" <- w245
        n174 = global write "加标回收状态全局变量.vi" "CODMn状态簇"(w245) -> ()
      }
    }
    n175 = flat-sequence {
      frame #0 {
        n176 = global read "质控内部交互全局.vi" "总磷通讯状态"() -> (→"总磷通讯":bool)
        n177 = global read "质控内部交互全局.vi" "总磷测量状态"() -> (w277:u16[])
        n178 = Index Array(array=w277) -> (element #1=w278:u16, element #2=w279:u16, element #3=w271:u16, element #4=w267:u16, element #5=w265:u16, element #6=w266:u16)  [unwired: 6 in]
        "总磷状态" <- w278
        n179 = Split Number(x=w267) -> (hi(x)=w269:u8, lo(x)=w268:u8)
        n180 = Bundle By Name(cluster=T1 {"步骤剩余时间"=0, "当前具体步骤"=enum."加标", " 当前流程"=enum."", "当前小步骤数"=0} ("氨氮状态簇"), "当前流程"=w269, "当前小步骤数"=w268, "步骤剩余时间"=w265, "当前具体步骤"=w266) -> (w263:T1)
        "总磷状态簇" <- w263
        n181 = global write "加标回收状态全局变量.vi" "总磷状态"(w278) -> ()
        n182 = Equal?(x=w279, y=u16 1) -> (x = y?=→"总磷传感器状态":bool)
        n183 = Equal?(x=w271, y=u16 1) -> (x = y?=→"总磷传感器故障报警":bool)
        n184 = Equal?(x=w271, y=u16 2) -> (x = y?=→"总磷柱塞泵故障报警":bool)
        n185 = global write "加标回收状态全局变量.vi" "总磷状态簇"(w263) -> ()
      }
    }
    n186 = flat-sequence {
      frame #0 {
        n187 = global read "质控内部交互全局.vi" "氨氮通讯状态"() -> (→"氨氮通讯":bool)
        n188 = global read "质控内部交互全局.vi" "氨氮测量状态"() -> (w295:u16[])
        n189 = Index Array(array=w295) -> (element #1=w296:u16, element #2=w298:u16, element #3=w289:u16, element #4=w285:u16, element #5=w283:u16, element #6=w284:u16)  [unwired: 6 in]
        "氨氮状态" <- w296
        n190 = Split Number(x=w285) -> (hi(x)=w287:u8, lo(x)=w286:u8)
        n191 = global write "加标回收状态全局变量.vi" "氨氮状态"(w296) -> ()
        n192 = Bundle By Name(cluster=T1 {"步骤剩余时间"=0, "当前具体步骤"=enum."加标", " 当前流程"=enum."", "当前小步骤数"=0} ("氨氮状态簇"), "当前流程"=w287, "当前小步骤数"=w286, "步骤剩余时间"=w283, "当前具体步骤"=w284) -> (w281:T1)
        "氨氮状态簇" <- w281
        n193 = Equal?(x=w298, y=u16 1) -> (x = y?=→"氨氮传感器状态":bool)
        n194 = Equal?(x=w289, y=u16 1) -> (x = y?=→"氨氮传感器故障报警":bool)
        n195 = Equal?(x=w289, y=u16 2) -> (x = y?=→"氨氮柱塞泵故障报警":bool)
        n196 = global write "加标回收状态全局变量.vi" "氨氮状态簇"(w281) -> ()
      }
    }
    n197 = Wait (ms)(milliseconds to wait=u32 1000 ("等待时间（毫秒）")) -> ()  [unwired: 1 out]
  }
  n198 = while {
    stop <- FALSE stop-if-true
    n199 = global read "质控测完标志全局 1.vi" "总磷总氮平行样测完标志"() -> (→"氨氮总磷平行样测完标志":bool)
    n200 = global read "水样浓度全局.vi" "CODCr加标前水样浓度"() -> (w356:dbl)
    n201 = local read "CODCr加标前水样浓度"() -> (w355:dbl)
    n202 = global read "质控测完标志全局 1.vi" "COD平行样测完标志"() -> (→"COD平行样测完标志":bool)
    n203 = global read "水样浓度全局.vi" "COD加标前水样浓度"() -> (w367:dbl)
    n204 = local read "总氮加标前水样浓度"() -> (w359:dbl)
    n205 = global read "水样浓度全局.vi" "氨氮加标前水样浓度"() -> (w371:dbl)
    n206 = global read "水样浓度全局.vi" "总磷加标前水样浓度"() -> (w369:dbl)
    n207 = local read "COD加标前水样浓度"() -> (w366:dbl)
    n208 = global read "水样浓度全局.vi" "总氮加标前水样浓度"() -> (w358:dbl)
    n209 = local read "氨氮加标前水样浓度"() -> (w370:dbl)
    n210 = local read "总磷加标前水样浓度"() -> (w368:dbl)
    n211 = Wait (ms)(milliseconds to wait=u32 1000 ("等待时间（毫秒）")) -> ()  [unwired: 1 out]
    n212 = Not Equal?(x=w371, y=w370) -> (x != y?=w365:bool)
    n213 = Not Equal?(x=w369, y=w368) -> (x != y?=w363:bool)
    n214 = Not Equal?(x=w367, y=w366) -> (x != y?=w362:bool)
    n215 = Not Equal?(x=w358, y=w359) -> (x != y?=w357:bool)
    n216 = Not Equal?(x=w356, y=w355) -> (x != y?=w354:bool)
    n217 = Compound Arithmetic op=OR ("复合运算")(w365, w363, w362, w357, w354) -> (w364:bool)
    n218 = case shown="真" w364 {
      frame False {
      }
      frame True {
        n219 = global read "水样浓度全局.vi" "CODCr加标前水样浓度"() -> (w374:dbl)
        n220 = global read "水样浓度全局.vi" "COD加标前水样浓度"() -> (w376:dbl)
        n221 = global read "水样浓度全局.vi" "总氮加标前水样浓度"() -> (w375:dbl)
        n222 = global read "水样浓度全局.vi" "总磷加标前水样浓度"() -> (w377:dbl)
        n223 = global read "水样浓度全局.vi" "氨氮加标前水样浓度"() -> (w378:dbl)
        n224 = property on="总氮加标前水样浓度" class="DigNum (严格)"("Val(Sgnl)"=w375) -> ()  [unwired: 2 in, 2 out]
        n225 = property on="CODCr加标前水样浓度" class="DigNum (严格)"("Val(Sgnl)"=w374) -> ()  [unwired: 2 in, 2 out]
        n226 = property on="COD加标前水样浓度" class="DigNum (严格)"("Val(Sgnl)"=w376) -> ()  [unwired: 2 in, 2 out]
        n227 = property on="总磷加标前水样浓度" class="DigNum (严格)"("Val(Sgnl)"=w377) -> ()  [unwired: 2 in, 2 out]
        n228 = property on="氨氮加标前水样浓度" class="DigNum (严格)"("Val(Sgnl)"=w378) -> ()  [unwired: 2 in, 2 out]
      }
    }
  }
  n229 = control-ref of="CODCr加标前水样浓度"() -> (w45:refnum<vi>)
  n230 = control-ref of="CODCr加标后水样浓度"() -> (w44:refnum<vi>)
  n231 = control-ref of="总氮加标水杯定容体积"() -> (w52:refnum<vi>)
  n232 = control-ref of="COD加标水杯定容体积"() -> (w67:refnum<vi>)
  n233 = control-ref of="总磷加标水杯定容体积"() -> (w76:refnum<vi>)
  n234 = control-ref of="氨氮加标水杯定容体积"() -> (w86:refnum<vi>)
  n235 = control-ref of="总氮加标前水样浓度"() -> (w54:refnum<vi>)
  n236 = control-ref of="总氮加标后水样浓度"() -> (w53:refnum<vi>)
  n237 = control-ref of="COD加标前水样浓度"() -> (w69:refnum<vi>)
  n238 = control-ref of="COD加标后水样浓度"() -> (w68:refnum<vi>)
  n239 = control-ref of="总磷加标前水样浓度"() -> (w78:refnum<vi>)
  n240 = control-ref of="总磷加标后水样浓度"() -> (w77:refnum<vi>)
  n241 = control-ref of="氨氮加标前水样浓度"() -> (w87:refnum<vi>)
  n242 = control-ref of="氨氮加标后水样浓度"() -> (w83:refnum<vi>)
  n243 = property on="窗格" class="Pane"("Origin"=T2 {"Horizontal"=0, "Vertical"=0} ("原点")) -> ()  [unwired: 2 in, 2 out]
  n244 = control-ref of="CODCr加标回收率"() -> (w40:refnum<vi>)
  n245 = control-ref of="CODCr母液浓度"() -> (w42:refnum<vi>)
  n246 = control-ref of="CODCr加标体积"() -> (w41:refnum<vi>)
  n247 = control-ref of="COD加标回收率"() -> (w64:refnum<vi>)
  n248 = control-ref of="总氮加标回收率"() -> (w49:refnum<vi>)
  n249 = control-ref of="总磷加标回收率"() -> (w74:refnum<vi>)
  n250 = control-ref of="氨氮加标回收率"() -> (w81:refnum<vi>)
  n251 = control-ref of="CODCr检出限"() -> (w46:refnum<vi>)
  n252 = control-ref of="总氮母液浓度"() -> (w51:refnum<vi>)
  n253 = control-ref of="总氮加标体积"() -> (w50:refnum<vi>)
  n254 = control-ref of="COD母液浓度"() -> (w66:refnum<vi>)
  n255 = control-ref of="COD加标体积"() -> (w65:refnum<vi>)
  n256 = control-ref of="总磷母液浓度"() -> (w75:refnum<vi>)
  n257 = control-ref of="总磷加标体积"() -> (w73:refnum<vi>)
  n258 = control-ref of="氨氮母液浓度"() -> (w85:refnum<vi>)
  n259 = control-ref of="氨氮加标体积"() -> (w82:refnum<vi>)
  n260 = control-ref of="CODCr量程"() -> (w47:refnum<vi>)
  n261 = control-ref of="总氮检出限"() -> (w55:refnum<vi>)
  n262 = control-ref of="COD检出限"() -> (w70:refnum<vi>)
  n263 = control-ref of="总磷检出限"() -> (w79:refnum<vi>)
  n264 = control-ref of="氨氮检出限"() -> (w88:refnum<vi>)
  n265 = control-ref of="总氮量程"() -> (w56:refnum<vi>)
  n266 = control-ref of="COD量程"() -> (w71:refnum<vi>)
  n267 = control-ref of="总磷量程"() -> (w80:refnum<vi>)
  n268 = control-ref of="氨氮量程"() -> (w89:refnum<vi>)
  n269 = Obtain Queue(name (unnamed)="质控单元" ("名称（未命名）"), element data type=cluster{"命令":string} {"命令"="启用模块"} ("元素")) -> (queue out=w3:refnum<queue>, error out=w2:errorcluster)  [unwired: 3 in, 1 out]
  n270 = while {
    tunnel: w3 -> [w384]
    tunnel: w2 -> [w383]
    stop <- FALSE stop-if-true
    # "通信入队列"
    n271 = Get Queue Status(queue=w384, error in (no error)=w383) -> (queue out=w381:refnum<queue>, error out=w380:errorcluster, # elements in queue=w382:i32)  [unwired: 1 in, 5 out]
    n272 = Equal To 0?(x=w382) -> (x = 0?=w379:bool)
    n273 = Wait (ms)(milliseconds to wait=u32 1000 ("等待时间（毫秒）")) -> ()  [unwired: 1 out]
    n274 = case shown="真" w379 {
      tunnel: w381 -> [_ w401]
      tunnel: w380 -> [_ w400]
      frame False {
      }
      frame True {
        n275 = local read "氨氮模块"() -> (w399:bool)
        n276 = case shown="真" w399 {
          tunnel: w401 -> [w427 w431]
          tunnel: w400 -> [w426 w430]
          tunnel: [w427 w429] -> w397
          tunnel: [w426 w428] -> w396
          frame False {
          }
          frame True {
            n277 = Enqueue Element(queue=w431, element=cluster{"命令":string} {"命令"="氨氮读取"} ("元素"), error in (no error)=w430) -> (queue out=w429:refnum<queue>, error out=w428:errorcluster)  [unwired: 1 in, 1 out]
          }
        }
        n278 = local read "总磷模块选择"() -> (w398:bool)
        n279 = case shown="真" w398 {
          tunnel: w397 -> [w420 w424]
          tunnel: w396 -> [w419 w423]
          tunnel: [w420 w422] -> w394
          tunnel: [w419 w421] -> w393
          frame False {
          }
          frame True {
            n280 = Enqueue Element(queue=w424, element=cluster{"命令":string} {"命令"="总磷读取"} ("元素"), error in (no error)=w423) -> (queue out=w422:refnum<queue>, error out=w421:errorcluster)  [unwired: 1 in, 1 out]
          }
        }
        n281 = local read "总氮模块选择"() -> (w395:bool)
        n282 = case shown="真" w395 {
          tunnel: w394 -> [w413 w417]
          tunnel: w393 -> [w412 w416]
          tunnel: [w413 w415] -> w391
          tunnel: [w412 w414] -> w390
          frame False {
          }
          frame True {
            n283 = Enqueue Element(queue=w417, element=cluster{"命令":string} {"命令"="总氮读取"} ("元素"), error in (no error)=w416) -> (queue out=w415:refnum<queue>, error out=w414:errorcluster)  [unwired: 1 in, 1 out]
          }
        }
        n284 = local read "CODMn选择"() -> (w392:bool)
        n285 = case shown="真" w392 {
          tunnel: w391 -> [w406 w410]
          tunnel: w390 -> [w405 w409]
          tunnel: [w406 w408] -> w388
          tunnel: [w405 w407] -> w387
          frame False {
          }
          frame True {
            n286 = Enqueue Element(queue=w410, element=cluster{"命令":string} {"命令"="CODMn读取"} ("元素"), error in (no error)=w409) -> (queue out=w408:refnum<queue>, error out=w407:errorcluster)  [unwired: 1 in, 1 out]
          }
        }
        n287 = local read "CODCr选择"() -> (w389:bool)
        n288 = case shown="真" w389 {
          tunnel: w388 -> [_ w403]
          tunnel: w387 -> [_ w402]
          frame False {
          }
          frame True {
            n289 = Enqueue Element(queue=w403, element=cluster{"命令":string} {"命令"="CODCr读取"} ("元素"), error in (no error)=w402) -> ()  [unwired: 1 in, 3 out]
          }
        }
      }
    }
  }
  n290 = while {
    shift-right: [w438] -> _
    shift-left: enum16{"待机", "启动COD", "COD测量中", "延时"}."待机" -> [w437]
    stop <- FALSE stop-if-true
    # "定时启动循环"
    n291 = global read "断电保存全局.vi" "定时控制"() -> (w433:T6)
    n292 = local read "定时启动"() -> (w435:bool)
    n293 = case shown="真" w435 {
      tunnel: w437 -> [_ w509]
      tunnel: [_ w508] -> w436
      frame False {
      }
      frame True {
        n294 = global read "断电保存全局.vi" "定时控制"() -> (w507:T6)
        n295 = Unbundle By Name(w507) -> ("周期设置类型"=w510:enum16{"定点启动", "间隔启动"}, "定时间隔"=w511:dbl, "24H周期设置"=w512:bool[])
        n296 = case shown="\"定点启动\", 默认" w510 {
          tunnel: w511 -> [_ w527]
          tunnel: w512 -> [w515 _]
          tunnel: w509 -> [w513 w530]
          tunnel: [w514 w525] -> w508
          frame "定点启动", Default {
            n297 = case shown="\"待机\", 默认" w513 {
              tunnel: w515 -> [w521 _]
              tunnel: [w516 _] -> w514
              frame "待机", Default {
                n298 = Get Date/Time In Seconds() -> (seconds since 1Jan1904=w523:timestamp)
                n299 = Seconds To Date/Time(time stamp (now)=w523) -> (date time rec=w522:T7)  [unwired: 1 in]
                n300 = Unbundle By Name(w522) -> ("时"=w520:i32, "分"=w519:i32)  [unwired: 1 out]
                n301 = Equal To 0?(x=w519) -> (x = 0?=w517:bool)
                n302 = Index Array(array=w521, index=w520) -> (element=w518:bool)
                n303 = Compound Arithmetic op=AND ("复合运算")(w518, w517) -> (w516:bool)
              }
              frame "启动COD" {
              }
            }
          }
          frame "间隔启动" {
            n304 = Multiply(x=w527, y=60.0) -> (x*y=w524:dbl)
            n305 = feedback #1(w524) -> (w529:dbl)
            n306 = case shown="\"待机\"" w530 {
              tunnel: w529 -> [_ w532]
              tunnel: [_ w531] -> w528
              frame Default {
              }
              frame "待机" {
                n307 = Increment(x=w532) -> (x+1=w531:dbl)
              }
            }
            n308 = feedback-in #1(w528) -> ()
            n309 = Greater Or Equal?(x=w528, y=w524) -> (x >= y?=w525:bool)
          }
        }
      }
    }
    n310 = Unbundle By Name(w433) -> ("定时功能启用"=w434:bool)
    n311 = local write "定时启动"(w434) -> ()
    n312 = Wait (ms)(milliseconds to wait=u32 1000 ("等待时间（毫秒）")) -> ()  [unwired: 1 out]
    n313 = case shown="\"启动COD\"" w437 {
      tunnel: [w441 w447 w455 enum16{"待机", "启动COD", "COD测量中", "延时"}."待机"] -> w438
      tunnel: w436 -> [w444 _ _ _]
      frame "待机", Default {
        n314 = Select(t=enum16{"待机", "启动COD", "COD测量中", "延时"}."启动COD", s=w444, f=enum16{"待机", "启动COD", "COD测量中", "延时"}."待机") -> (s? t:f=w441:enum16{"待机", "启动COD", "COD测量中", "延时"})
      }
      frame "启动COD" {
        n315 = global read "断电保存全局.vi" "定时控制"() -> (w445:T6)
        n316 = Unbundle By Name(w445) -> ("模块选择"=w446:T8)
        n317 = flat-sequence {
          tunnel: w446 -> [w453]
          tunnel: [enum16{"待机", "启动COD", "COD测量中", "延时"}."COD测量中"] -> w447
          frame #0 {
            n318 = Unbundle By Name(w453) -> ("氨氮"=w452:bool, "总磷"=w451:bool, "总氮"=w450:bool, "CODMn"=w449:bool, "CODCr"=w448:bool)
            n319 = case shown="真" w452 {
              frame False {
              }
              frame True {
                n320 = call "氨氮加标回收 (子VI).vi"() -> ()  [unwired: 12 in]
              }
            }
            n321 = case shown="真" w451 {
              frame False {
              }
              frame True {
                n322 = call "总磷加标回收 (子VI).vi"() -> ()  [unwired: 12 in]
              }
            }
            n323 = case shown="真" w450 {
              frame False {
              }
              frame True {
                n324 = call "总氮加标回收 (子VI).vi"() -> ()  [unwired: 12 in]
              }
            }
            n325 = case shown="真" w449 {
              frame False {
              }
              frame True {
                n326 = call "CODMn加标回收(子VI).vi"() -> ()  [unwired: 12 in]
              }
            }
            n327 = case shown="真" w448 {
              frame False {
              }
              frame True {
                n328 = call "CODCr加标回收(子VI).vi"() -> ()  [unwired: 12 in]
              }
            }
          }
          frame #1 {
          }
        }
      }
      frame "COD测量中" {
        n329 = global read "断电保存全局.vi" "定时控制"() -> (w469:T6)
        n330 = Unbundle By Name(w469) -> ("模块选择"=w468:T8)
        n331 = Unbundle By Name(w468) -> ("氨氮"=w460:bool, "总磷"=w459:bool, "总氮"=w458:bool, "CODMn"=w457:bool, "CODCr"=w456:bool)
        n332 = case shown="真" w460 {
          tunnel: [TRUE w503] -> w461
          frame False {
          }
          frame True {
            # "氨氮测完"
            n333 = global read "质控测完标志全局 1.vi" "氨氮质控流程中"() -> (w505:bool)
            n334 = global read "加标回收状态全局变量.vi" "氨氮状态"() -> (w502:u16)
            n335 = Equal To 0?(x=w502) -> (x = 0?=w501:bool)
            n336 = Not(x=w505) -> (.not. x?=w504:bool)
            n337 = And(x=w501, y=w504) -> (x .and. y?=w503:bool)
          }
        }
        n338 = case shown="真" w459 {
          tunnel: [TRUE w497] -> w462
          frame False {
          }
          frame True {
            # "总磷测完"
            n339 = global read "质控测完标志全局 1.vi" "总磷质控流程中"() -> (w499:bool)
            n340 = global read "加标回收状态全局变量.vi" "总磷状态"() -> (w496:u16)
            n341 = Equal To 0?(x=w496) -> (x = 0?=w495:bool)
            n342 = Not(x=w499) -> (.not. x?=w498:bool)
            n343 = And(x=w495, y=w498) -> (x .and. y?=w497:bool)
          }
        }
        n344 = case shown="真" w458 {
          tunnel: [TRUE w491] -> w463
          frame False {
          }
          frame True {
            # "总氮测完"
            n345 = global read "质控测完标志全局 1.vi" "总氮质控流程中"() -> (w493:bool)
            n346 = global read "加标回收状态全局变量.vi" "总氮状态"() -> (w490:u16)
            n347 = Equal To 0?(x=w490) -> (x = 0?=w489:bool)
            n348 = Not(x=w493) -> (.not. x?=w492:bool)
            n349 = And(x=w489, y=w492) -> (x .and. y?=w491:bool)
          }
        }
        n350 = case shown="真" w457 {
          tunnel: [TRUE w485] -> w464
          frame False {
          }
          frame True {
            # "CODMn测完"
            n351 = global read "质控测完标志全局 1.vi" "COD质控流程中"() -> (w487:bool)
            n352 = global read "加标回收状态全局变量.vi" "COD状态"() -> (w484:u16)
            n353 = Equal To 0?(x=w484) -> (x = 0?=w483:bool)
            n354 = Not(x=w487) -> (.not. x?=w486:bool)
            n355 = And(x=w483, y=w486) -> (x .and. y?=w485:bool)
          }
        }
        n356 = case shown="真" w456 {
          tunnel: [TRUE w479] -> w465
          frame False {
          }
          frame True {
            # "CODCr测完"
            n357 = global read "质控测完标志全局 1.vi" "CODCr质控流程中"() -> (w481:bool)
            n358 = global read "加标回收状态全局变量.vi" "CODCr状态"() -> (w478:u16)
            n359 = Equal To 0?(x=w478) -> (x = 0?=w477:bool)
            n360 = Not(x=w481) -> (.not. x?=w480:bool)
            n361 = And(x=w477, y=w480) -> (x .and. y?=w479:bool)
          }
        }
        n362 = Compound Arithmetic op=AND ("复合运算")(w461, w462, w463, w464, w465) -> (w466:bool)
        n363 = flat-sequence {
          tunnel: [w471] -> w467
          tunnel: w466 -> [w470]
          tunnel: [w475] -> w455
          tunnel: w467 -> [w475]
          frame #0 {
            n364 = Select(t=enum16{"待机", "启动COD", "COD测量中", "延时"}."延时", s=w470, f=enum16{"待机", "启动COD", "COD测量中", "延时"}."COD测量中") -> (s? t:f=w471:enum16{"待机", "启动COD", "COD测量中", "延时"})
          }
          frame #1 {
            n365 = Wait (ms)(milliseconds to wait=u32 5000 ("等待时间（毫秒）")) -> ()  [unwired: 1 out]
          }
        }
      }
      frame "延时" {
      }
    }
  }
  n366 = property class="VI"(reference=w31) -> ("Name"=w32:string)  [unwired: 1 in, 2 out]
  n367 = Build Array(w47, w46, w45, w44, w43, w42, w41, w40) -> (w39:refnum<vi>[])
  n368 = Build Array(w56, w55, w54, w53, w52, w51, w50, w49) -> (w48:refnum<vi>[])
  n369 = Build Array(w71, w70, w69, w68, w67, w66, w65, w64) -> (w63:refnum<vi>[])
  n370 = Build Array(w80, w79, w78, w77, w76, w75, w73, w74) -> (w72:refnum<vi>[])
  n371 = Build Array(w89, w88, w87, w83, w86, w85, w82, w81) -> (w84:refnum<vi>[])
  n372 = property class="VI"(reference=w18) -> ("Name"=w17:string)  [unwired: 1 in, 2 out]
  n373 = Obtain Notifier(name (unnamed)="采配水Process" ("名称（未命名）"), notification data type=FALSE) -> (notifier out=w60:refnum<notifier>)  [unwired: 2 in, 2 out]
  n374 = Obtain Queue(name (unnamed)="采配水" ("名称（未命名）"), element data type=cluster{"命令":string, "数据":variant} {"命令"="", "数据"=variant}) -> (queue out=w57:refnum<queue>)  [unwired: 3 in, 2 out]
  n375 = Obtain Queue(name (unnamed)="质控单元" ("名称（未命名）"), element data type=cluster{"命令":string} {"命令"="启用模块"} ("元素")) -> (queue out=w28:refnum<queue>, error out=w27:errorcluster)  [unwired: 3 in, 1 out]
  n376 = control-ref of="CODCr加标后水样浓度"() -> (w6:refnum<vi>)
  n377 = property class="VI"(reference=w26) -> ("Name"=w25:string)  [unwired: 1 in, 2 out]
  n378 = control-ref of="总氮加标后水样浓度"() -> (w10:refnum<vi>)
  n379 = control-ref of="COD加标后水样浓度"() -> (w7:refnum<vi>)
  n380 = control-ref of="氨氮加标后水样浓度"() -> (w9:refnum<vi>)
  n381 = control-ref of="总磷加标后水样浓度"() -> (w8:refnum<vi>)
  n382 = Open VI Reference(type specifier VI Refnum (for type only)=refnum<vi> refnum, vi path=w32, options=128 ("选项")) -> (vi reference=w34:refnum<vi>, error out=w36:errorcluster)  [unwired: 3 in]
  n383 = Open VI Reference(type specifier VI Refnum (for type only)=refnum<vi> refnum, vi path=w17, options=128 ("选项")) -> (vi reference=w15:refnum<vi>, error out=w13:errorcluster)  [unwired: 3 in]
  n384 = while {
    tunnel: w84 -> [w541]
    tunnel: w72 -> [w540]
    tunnel: w63 -> [w535]
    tunnel: w60 -> [w539]
    tunnel: w57 -> [w538]
    tunnel: w48 -> [w537]
    tunnel: w39 -> [w536]
    tunnel: w28 -> [w534]
    tunnel: w27 -> [w533]
    stop <- FALSE stop-if-true
    # "氨氮站号是1，总磷站号是2，总氮站号3，CODMn站号是4，CODCr站号是5"
    n385 = event shown="[23] \"定时启动\": 值改变" {
      selector: _ -> [_ _ _ _ _ _ _ _ _ _ _ _ _ _ _ _ _ _ _ _ _ _ _ _ _ _]
      dyn-events: _ -> [_ _ _ _ _ _ _ _ _ _ _ _ _ _ _ _ _ _ _ _ _ _ _ _ _ _]
      timeout: _ -> [_ _ _ _ _ _ _ _ _ _ _ _ _ _ _ _ _ _ _ _ _ _ _ _ _ _]
      tunnel: w541 -> [_ _ _ _ _ _ _ _ _ _ w642 _ _ _ _ _ _ _ _ _ _ _ _ _ _ _]
      tunnel: w540 -> [_ _ _ _ _ _ _ _ _ _ _ w656 _ _ _ _ _ _ _ _ _ _ _ _ _ _]
      tunnel: w535 -> [_ _ _ _ _ _ _ _ _ _ _ _ _ w694 _ _ _ _ _ _ _ _ _ _ _ _]
      tunnel: w539 -> [_ _ _ _ _ _ _ _ _ _ _ _ _ _ _ _ _ _ _ w780 _ w847 w863 _ _ _]
      tunnel: w538 -> [_ _ _ _ _ _ _ _ _ _ _ _ _ _ _ _ _ _ _ _ _ _ w864 _ _ _]
      tunnel: w537 -> [_ _ _ _ _ _ _ _ _ _ _ _ w674 _ _ _ _ _ _ _ _ _ _ _ _ _]
      tunnel: w536 -> [_ _ _ _ _ _ _ _ _ _ _ _ _ _ w712 _ _ _ _ _ _ _ _ _ _ _]
      tunnel: w534 -> [_ _ _ _ _ _ _ _ _ _ _ _ _ _ _ _ _ w736 w770 _ _ _ _ _ _ _]
      tunnel: w533 -> [_ _ _ _ _ _ _ _ _ _ _ _ _ _ _ _ _ w735 w769 _ _ _ _ _ _ _]
      event Timeout {
        n386 = event-data() -> ()  [unwired: 1 in, 3 out]
      }
      event "氨氮量程", "氨氮检出限", "氨氮加标前水样浓度", "氨氮加标水杯定容体积", "氨氮母液浓度", "氨氮加标后水样浓度": Mouse Down {
        n387 = event-data() -> ("CtlRef"=w546:refnum<vi>)  [unwired: 1 in, 7 out]
        n388 = property class="DigNum (严格)"(reference=w546) -> (reference out=w544:refnum<vi>, "Value"=w545:dbl)  [unwired: 1 in, 1 out]
        n389 = call "数字键盘.vi"("OldNumber"=w545) -> ("NewNumber"=w543:sgl)
        n390 = property class="DigNum (严格)"(reference=w544, "Val(Sgnl)"=w543) -> ()  [unwired: 1 in, 2 out]
      }
      event "总磷母液浓度", "总磷加标水杯定容体积", "总磷加标后水样浓度", "总磷加标前水样浓度", "总磷检出限", "总磷量程": Mouse Down {
        n391 = event-data() -> ("CtlRef"=w550:refnum<vi>)  [unwired: 1 in, 7 out]
        n392 = property class="DigNum (严格)"(reference=w550) -> (reference out=w548:refnum<vi>, "Value"=w549:dbl)  [unwired: 1 in, 1 out]
        n393 = call "数字键盘.vi"("OldNumber"=w549) -> ("NewNumber"=w547:sgl)
        n394 = property class="DigNum (严格)"(reference=w548, "Val(Sgnl)"=w547) -> ()  [unwired: 1 in, 2 out]
      }
      event "总氮母液浓度", "总氮加标水杯定容体积", "总氮加标后水样浓度", "总氮加标前水样浓度", "总氮检出限", "总氮量程": Mouse Down {
        n395 = event-data() -> ("CtlRef"=w554:refnum<vi>)  [unwired: 1 in, 7 out]
        n396 = property class="DigNum (严格)"(reference=w554) -> (reference out=w552:refnum<vi>, "Value"=w553:dbl)  [unwired: 1 in, 1 out]
        n397 = call "数字键盘.vi"("OldNumber"=w553) -> ("NewNumber"=w551:sgl)
        n398 = property class="DigNum (严格)"(reference=w552, "Val(Sgnl)"=w551) -> ()  [unwired: 1 in, 2 out]
      }
      event "COD母液浓度", "COD加标水杯定容体积", "COD加标后水样浓度", "COD加标前水样浓度", "COD检出限", "COD量程": Mouse Down {
        n399 = event-data() -> ("CtlRef"=w558:refnum<vi>)  [unwired: 1 in, 7 out]
        n400 = property class="DigNum (严格)"(reference=w558) -> (reference out=w556:refnum<vi>, "Value"=w557:dbl)  [unwired: 1 in, 1 out]
        n401 = call "数字键盘.vi"("OldNumber"=w557) -> ("NewNumber"=w555:sgl)
        n402 = property class="DigNum (严格)"(reference=w556, "Val(Sgnl)"=w555) -> ()  [unwired: 1 in, 2 out]
      }
      event "CODCr检出限", "CODCr量程", "CODCr加标前水样浓度", "CODCr加标后水样浓度", "CODCr加标水杯定容体积", "CODCr母液浓度": Mouse Down {
        n403 = event-data() -> ("CtlRef"=w559:refnum<vi>)  [unwired: 1 in, 7 out]
        n404 = property class="DigNum (严格)"(reference=w559) -> (reference out=w561:refnum<vi>, "Value"=w562:dbl)  [unwired: 1 in, 1 out]
        n405 = call "数字键盘.vi"("OldNumber"=w562) -> ("NewNumber"=w560:sgl)
        n406 = property class="DigNum (严格)"(reference=w561, "Val(Sgnl)"=w560) -> ()  [unwired: 1 in, 2 out]
      }
      event "背隙补偿步数", "背隙补偿步数 2", "背隙补偿步数 3": Mouse Down {
        n407 = event-data() -> ("CtlRef"=w566:refnum<vi>)  [unwired: 1 in, 7 out]
        n408 = property class="DigNum (严格)"(reference=w566) -> (reference out=w565:refnum<vi>, "Value"=w564:i32)  [unwired: 1 in, 1 out]
        n409 = call "数字键盘.vi"("OldNumber"=w564) -> ("NewNumber"=w563:sgl)
        n410 = property class="DigNum (严格)"(reference=w565, "Val(Sgnl)"=w563) -> ()  [unwired: 1 in, 2 out]
      }
      event "背隙补偿步数", "背隙补偿步数 2", "背隙补偿步数 3": Value Change {
        w575 = "质控背隙补偿" ("section")
        n411 = event-data() -> ()  [unwired: 1 in, 6 out]
        n412 = call <vilib>:"Application Directory.vi"() -> ("Application Directory"=w582:path)
        n413 = Build Path(base path=w582, name or relative path="data\\Set.ini" ("名称或相对路径")) -> (appended path=w580:path)
        n414 = call <vilib>:"Open Config Data.vi"("configuration file path"=w580) -> ("error out"=w578:errorcluster, "refnum"=w579:T3)  [unwired: 8 in, 1 out]
        n415 = call-poly <vilib>:"Write Key.vi"("section"=w575, "error in (no error)"=w578, "value"="背隙补偿步数", "key"="背隙值1", "refnum"=w579) -> ("error out"=w569:errorcluster, "refnum out"=w572:T3)  [unwired: 4 in, 1 out]
        n416 = call-poly <vilib>:"Write Key.vi"("section"=w575, "error in (no error)"=w569, "value"="背隙补偿步数 2", "key"="背隙值2", "refnum"=w572) -> ("error out"=w570:errorcluster, "refnum out"=w571:T3)  [unwired: 4 in, 1 out]
        n417 = call-poly <vilib>:"Write Key.vi"("section"=w575, "error in (no error)"=w570, "value"="背隙补偿步数 3", "key"="背隙值3", "refnum"=w571) -> ()  [unwired: 4 in, 3 out]
      }
      event "氨氮模块", "总磷模块选择", "CODMn选择", "CODCr选择", "总氮模块选择": Value Change {
        w589 = "质控模块选择" ("section")
        n418 = event-data() -> ()  [unwired: 1 in, 6 out]
        n419 = call <vilib>:"Application Directory.vi"() -> ("Application Directory"=w609:path)
        n420 = Build Path(base path=w609, name or relative path="data\\Set.ini" ("名称或相对路径")) -> (appended path=w607:path)
        n421 = local read "氨氮模块"() -> (w599:bool)
        n422 = call <vilib>:"Open Config Data.vi"("configuration file path"=w607) -> ("error out"=w605:errorcluster, "refnum"=w606:T3)  [unwired: 8 in, 1 out]
        n423 = local read "总磷模块选择"() -> (w598:bool)
        n424 = call-poly <vilib>:"Write Key.vi"("section"=w589, "error in (no error)"=w605, "value"=w599, "key"="模块1" ("section"), "refnum"=w606) -> ("error out"=w603:errorcluster, "refnum out"=w604:T3)  [unwired: 4 in, 1 out]
        n425 = local read "总氮模块选择"() -> (w584:bool)
        n426 = call-poly <vilib>:"Write Key.vi"("section"=w589, "error in (no error)"=w603, "value"=w598, "key"="模块2" ("section"), "refnum"=w604) -> ("error out"=w587:errorcluster, "refnum out"=w588:T3)  [unwired: 4 in, 1 out]
        n427 = local read "CODMn选择"() -> (w597:bool)
        n428 = call-poly <vilib>:"Write Key.vi"("section"=w589, "error in (no error)"=w587, "value"=w584, "key"="模块3" ("section"), "refnum"=w588) -> ("error out"=w585:errorcluster, "refnum out"=w586:T3)  [unwired: 4 in, 1 out]
        n429 = local read "CODCr选择"() -> (w591:bool)
        n430 = call-poly <vilib>:"Write Key.vi"("section"=w589, "error in (no error)"=w585, "value"=w597, "key"="模块4" ("section"), "refnum"=w586) -> ("error out"=w594:errorcluster, "refnum out"=w595:T3)  [unwired: 4 in, 1 out]
        n431 = call-poly <vilib>:"Write Key.vi"("section"=w589, "error in (no error)"=w594, "value"=w591, "key"="模块5" ("section"), "refnum"=w595) -> ("error out"=w592:errorcluster, "refnum out"=w593:T3)  [unwired: 4 in, 1 out]
        n432 = call <vilib>:"Close Config Data.vi"("error in (no error)"=w592, "refnum"=w593) -> ("error out"=w583:errorcluster)  [unwired: 8 in, 1 out]
        n433 = call <vilib>:"Clear Errors.vi"("error in (no error)"=w583) -> ()  [unwired: 5 in, 2 out]
      }
      event "氨氮量程选择", "总氮量程选择", "总磷量程选择", "CODMn量程选择", "CODCr量程选择": Value Change {
        w616 = "质控模块量程选择" ("section")
        n434 = event-data() -> ()  [unwired: 1 in, 6 out]
        n435 = call <vilib>:"Application Directory.vi"() -> ("Application Directory"=w635:path)
        n436 = Build Path(base path=w635, name or relative path="data\\Set.ini" ("名称或相对路径")) -> (appended path=w633:path)
        n437 = local read "氨氮量程选择"() -> (w620:enum32{"H", "L", "AUTO"})
        n438 = call <vilib>:"Open Config Data.vi"("configuration file path"=w633) -> ("error out"=w631:errorcluster, "refnum"=w632:T3)  [unwired: 8 in, 1 out]
        n439 = local read "总氮量程选择"() -> (w619:enum32{"H", "L", "AUTO"})
        n440 = call-poly <vilib>:"Write Key.vi"("section"=w616, "error in (no error)"=w631, "value"=w620, "key"="氨氮" ("section"), "refnum"=w632) -> ("error out"=w629:errorcluster, "refnum out"=w630:T3)  [unwired: 4 in, 1 out]
        n441 = local read "总磷量程选择"() -> (w618:enum32{"H", "L", "AUTO"})
        n442 = call-poly <vilib>:"Write Key.vi"("section"=w616, "error in (no error)"=w629, "value"=w619, "key"="总氮" ("section"), "refnum"=w630) -> ("error out"=w627:errorcluster, "refnum out"=w628:T3)  [unwired: 4 in, 1 out]
        n443 = local read "CODMn量程选择"() -> (w617:enum32{"H", "L", "AUTO"})
        n444 = call-poly <vilib>:"Write Key.vi"("section"=w616, "error in (no error)"=w627, "value"=w618, "key"="总磷" ("section"), "refnum"=w628) -> ("error out"=w622:errorcluster, "refnum out"=w623:T3)  [unwired: 4 in, 1 out]
        n445 = local read "CODCr量程选择"() -> (w610:enum32{"H", "L", "AUTO"})
        n446 = call-poly <vilib>:"Write Key.vi"("section"=w616, "error in (no error)"=w622, "value"=w617, "key"="CODMn" ("section"), "refnum"=w623) -> ("error out"=w612:errorcluster, "refnum out"=w615:T3)  [unwired: 4 in, 1 out]
        n447 = call-poly <vilib>:"Write Key.vi"("section"=w616, "error in (no error)"=w612, "value"=w610, "key"="CODCr" ("section"), "refnum"=w615) -> ("error out"=w613:errorcluster, "refnum out"=w614:T3)  [unwired: 4 in, 1 out]
        n448 = call <vilib>:"Close Config Data.vi"("error in (no error)"=w613, "refnum"=w614) -> ()  [unwired: 8 in, 2 out]
      }
      event "氨氮量程", "氨氮检出限", "氨氮加标前水样浓度", "氨氮母液浓度", "氨氮加标水杯定容体积", "氨氮加标后水样浓度": Value Change {
        n449 = event-data() -> ()  [unwired: 1 in, 6 out]
        n450 = for {
          tunnel: w642 -> [w654] mode=indexing
          tunnel: [w653] -> w651 mode=indexing
          n451 = property class="DigNum (严格)"(reference=w654) -> ("Value"=w653:dbl)  [unwired: 1 in, 2 out]
        }
        n452 = Index Array(array=w651) -> (element #1=w650:dbl, element #2=w649:dbl, element #3=w636:dbl, element #4=w648:dbl, element #5=w647:dbl, element #6=w645:dbl)  [unwired: 6 in]
        n453 = global write "水样浓度全局.vi" "氨氮加标前水样浓度"(w636) -> ()
        n454 = Bundle By Name(cluster=T4 {"量程"=0.0, "检出限"=0.0, "加标前水样浓度"=0.0, "加标后水样浓度"=0.0, "加标水杯定容体积"=0.0, "加标母液浓度"=0.0, "加标体积"=0.0, "加标回收率"=0.0} ("参数"), "量程"=w650, "检出限"=w649, "加标前水样浓度"=w636, "加标后水样浓度"=w648, "加标水杯定容体积"=w647, "加标母液浓度"=w645) -> (w644:T4)
        n455 = call "加标回收率计算.vi"("参数"=w644) -> ("参数 out"=w643:T4)  [unwired: 10 in]
        n456 = call "质控参数保存.vi"("section"="氨氮质控参数", "参数"=w643) -> ()  [unwired: 9 in, 1 out]
        n457 = Unbundle By Name(w643) -> ("加标体积"=w637:dbl, "加标回收率"=w638:dbl)
        n458 = Index Array(array=w642, index #1=6 ("索引")) -> (element #1=w641:refnum<vi>, element #2=w639:refnum<vi>)  [unwired: 1 in]
        n459 = property class="DigNum (严格)"(reference=w641, "Value"=w637) -> ()  [unwired: 1 in, 2 out]
        n460 = property class="DigNum (严格)"(reference=w639, "Value"=w638) -> ()  [unwired: 1 in, 2 out]
      }
      event "总磷母液浓度", "总磷加标水杯定容体积", "总磷加标后水样浓度", "总磷加标前水样浓度", "总磷检出限", "总磷量程": Value Change {
        n461 = event-data() -> ()  [unwired: 1 in, 6 out]
        n462 = for {
          tunnel: w656 -> [w673] mode=indexing
          tunnel: [w672] -> w670 mode=indexing
          n463 = property class="DigNum (严格)"(reference=w673) -> ("Value"=w672:dbl)  [unwired: 1 in, 2 out]
        }
        n464 = Index Array(array=w670) -> (element #1=w669:dbl, element #2=w668:dbl, element #3=w655:dbl, element #4=w667:dbl, element #5=w666:dbl, element #6=w664:dbl)  [unwired: 6 in]
        n465 = global write "水样浓度全局.vi" "总磷加标前水样浓度"(w655) -> ()
        n466 = Bundle By Name(cluster=T4 {"量程"=0.0, "检出限"=0.0, "加标前水样浓度"=0.0, "加标后水样浓度"=0.0, "加标水杯定容体积"=0.0, "加标母液浓度"=0.0, "加标体积"=0.0, "加标回收率"=0.0} ("参数"), "量程"=w669, "检出限"=w668, "加标前水样浓度"=w655, "加标后水样浓度"=w667, "加标水杯定容体积"=w666, "加标母液浓度"=w664) -> (w663:T4)
        n467 = call "加标回收率计算.vi"("参数"=w663) -> ("参数 out"=w662:T4)  [unwired: 10 in]
        n468 = call "质控参数保存.vi"("section"="总磷质控参数", "参数"=w662) -> ()  [unwired: 9 in, 1 out]
        n469 = Unbundle By Name(w662) -> ("加标体积"=w659:dbl, "加标回收率"=w657:dbl)
        n470 = Index Array(array=w656, index #1=6 ("索引")) -> (element #1=w661:refnum<vi>, element #2=w658:refnum<vi>)  [unwired: 1 in]
        n471 = property class="DigNum (严格)"(reference=w661, "Value"=w659) -> ()  [unwired: 1 in, 2 out]
        n472 = property class="DigNum (严格)"(reference=w658, "Value"=w657) -> ()  [unwired: 1 in, 2 out]
      }
      event "总氮量程", "总氮检出限", "总氮加标前水样浓度", "总氮加标后水样浓度", "总氮加标水杯定容体积", "总氮母液浓度": Value Change {
        n473 = event-data() -> ()  [unwired: 1 in, 6 out]
        n474 = for {
          tunnel: w674 -> [w692] mode=indexing
          tunnel: [w691] -> w689 mode=indexing
          n475 = property class="DigNum (严格)"(reference=w692) -> ("Value"=w691:dbl)  [unwired: 1 in, 2 out]
        }
        n476 = Index Array(array=w689) -> (element #1=w688:dbl, element #2=w687:dbl, element #3=w675:dbl, element #4=w686:dbl, element #5=w685:dbl, element #6=w683:dbl)  [unwired: 6 in]
        n477 = global write "水样浓度全局.vi" "总氮加标前水样浓度"(w675) -> ()
        n478 = Bundle By Name(cluster=T4 {"量程"=0.0, "检出限"=0.0, "加标前水样浓度"=0.0, "加标后水样浓度"=0.0, "加标水杯定容体积"=0.0, "加标母液浓度"=0.0, "加标体积"=0.0, "加标回收率"=0.0} ("参数"), "量程"=w688, "检出限"=w687, "加标前水样浓度"=w675, "加标后水样浓度"=w686, "加标水杯定容体积"=w685, "加标母液浓度"=w683) -> (w682:T4)
        n479 = call "加标回收率计算.vi"("参数"=w682) -> ("参数 out"=w681:T4)  [unwired: 10 in]
        n480 = call "质控参数保存.vi"("section"="总氮质控参数", "参数"=w681) -> ()  [unwired: 9 in, 1 out]
        n481 = Unbundle By Name(w681) -> ("加标体积"=w678:dbl, "加标回收率"=w676:dbl)
        n482 = Index Array(array=w674, index #1=6 ("索引")) -> (element #1=w680:refnum<vi>, element #2=w677:refnum<vi>)  [unwired: 1 in]
        n483 = property class="DigNum (严格)"(reference=w680, "Value"=w678) -> ()  [unwired: 1 in, 2 out]
        n484 = property class="DigNum (严格)"(reference=w677, "Value"=w676) -> ()  [unwired: 1 in, 2 out]
      }
      event "COD母液浓度", "COD加标水杯定容体积", "COD加标后水样浓度", "COD加标前水样浓度", "COD检出限", "COD量程": Value Change {
        n485 = event-data() -> ()  [unwired: 1 in, 6 out]
        n486 = for {
          tunnel: w694 -> [w711] mode=indexing
          tunnel: [w710] -> w708 mode=indexing
          n487 = property class="DigNum (严格)"(reference=w711) -> ("Value"=w710:dbl)  [unwired: 1 in, 2 out]
        }
        n488 = Index Array(array=w708) -> (element #1=w707:dbl, element #2=w706:dbl, element #3=w693:dbl, element #4=w705:dbl, element #5=w704:dbl, element #6=w702:dbl)  [unwired: 6 in]
        n489 = global write "水样浓度全局.vi" "COD加标前水样浓度"(w693) -> ()
        n490 = Bundle By Name(cluster=T4 {"量程"=0.0, "检出限"=0.0, "加标前水样浓度"=0.0, "加标后水样浓度"=0.0, "加标水杯定容体积"=0.0, "加标母液浓度"=0.0, "加标体积"=0.0, "加标回收率"=0.0} ("参数"), "量程"=w707, "检出限"=w706, "加标前水样浓度"=w693, "加标后水样浓度"=w705, "加标水杯定容体积"=w704, "加标母液浓度"=w702) -> (w701:T4)
        n491 = call "加标回收率计算.vi"("参数"=w701) -> ("参数 out"=w700:T4)  [unwired: 10 in]
        n492 = call "质控参数保存.vi"("section"="COD质控参数", "参数"=w700) -> ()  [unwired: 9 in, 1 out]
        n493 = Unbundle By Name(w700) -> ("加标体积"=w697:dbl, "加标回收率"=w695:dbl)
        n494 = Index Array(array=w694, index #1=6 ("索引")) -> (element #1=w699:refnum<vi>, element #2=w696:refnum<vi>)  [unwired: 1 in]
        n495 = property class="DigNum (严格)"(reference=w699, "Value"=w697) -> ()  [unwired: 1 in, 2 out]
        n496 = property class="DigNum (严格)"(reference=w696, "Value"=w695) -> ()  [unwired: 1 in, 2 out]
      }
      event "CODCr母液浓度", "CODCr加标水杯定容体积", "CODCr加标前水样浓度", "CODCr检出限", "CODCr量程", "CODCr加标后水样浓度": Value Change {
        n497 = event-data() -> ()  [unwired: 1 in, 6 out]
        n498 = for {
          tunnel: w712 -> [w730] mode=indexing
          tunnel: [w729] -> w727 mode=indexing
          n499 = property class="DigNum (严格)"(reference=w730) -> ("Value"=w729:dbl)  [unwired: 1 in, 2 out]
        }
        n500 = Index Array(array=w727) -> (element #1=w726:dbl, element #2=w725:dbl, element #3=w713:dbl, element #4=w724:dbl, element #5=w723:dbl, element #6=w721:dbl)  [unwired: 6 in]
        n501 = global write "水样浓度全局.vi" "CODCr加标前水样浓度"(w713) -> ()
        n502 = Bundle By Name(cluster=T4 {"量程"=0.0, "检出限"=0.0, "加标前水样浓度"=0.0, "加标后水样浓度"=0.0, "加标水杯定容体积"=0.0, "加标母液浓度"=0.0, "加标体积"=0.0, "加标回收率"=0.0} ("参数"), "量程"=w726, "检出限"=w725, "加标前水样浓度"=w713, "加标后水样浓度"=w724, "加标水杯定容体积"=w723, "加标母液浓度"=w721) -> (w720:T4)
        n503 = call "加标回收率计算.vi"("参数"=w720) -> ("参数 out"=w719:T4)  [unwired: 10 in]
        n504 = call "质控参数保存.vi"("section"="CODCr质控参数", "参数"=w719) -> ()  [unwired: 9 in, 1 out]
        n505 = Unbundle By Name(w719) -> ("加标体积"=w716:dbl, "加标回收率"=w714:dbl)
        n506 = Index Array(array=w712, index #1=6 ("索引")) -> (element #1=w718:refnum<vi>, element #2=w715:refnum<vi>)  [unwired: 1 in]
        n507 = property class="DigNum (严格)"(reference=w718, "Value"=w716) -> ()  [unwired: 1 in, 2 out]
        n508 = property class="DigNum (严格)"(reference=w715, "Value"=w714) -> ()  [unwired: 1 in, 2 out]
      }
      event "手动调试": Value Change {
        n509 = event-data() -> ()  [unwired: 1 in, 6 out]
        n510 = call "手动调试界面.vi"() -> ()  [unwired: 16 in]
      }
      event "柱塞泵调试": Value Change {
        n511 = event-data() -> ()  [unwired: 1 in, 6 out]
        n512 = call "柱塞泵调试界面.vi"() -> ()  [unwired: 16 in]
      }
      event "打开串口": Value Change {
        n513 = event-data() -> ()  [unwired: 1 in, 6 out]
        n514 = global read "断电保存全局.vi" "MB通信方式选择"() -> (w731:enum16{"串口", "TCP"})
        n515 = global read "断电保存全局.vi" "VISA Resource"() -> (w732:refnum<visa-resource-name>)
        n516 = global read "断电保存全局.vi" "PORT"() -> (w733:string)
        n517 = global read "断电保存全局.vi" "IP"() -> (w734:string)
        n518 = call "串口配置.vi"("PORT"=w733, "IP"=w734, "MB通信方式选择"=w731, "请选择串口:"=w732) -> ("PORT 2"=w738:string, "IP 2"=w739:string, "确认 2"=w741:bool, "VISA资源名称 2"=w740:refnum<visa-resource-name>, "MB通信方式选择 2"=w737:enum16{"串口", "TCP"})  [unwired: 3 in]
        n519 = case shown="真" w741 {
          tunnel: w740 -> [_ w747]
          tunnel: w736 -> [_ w746]
          tunnel: w739 -> [_ w745]
          tunnel: w738 -> [_ w744]
          tunnel: w737 -> [_ w743]
          tunnel: w735 -> [_ w742]
          frame False {
          }
          frame True {
            n520 = flat-sequence {
              tunnel: w747 -> [w751]
              tunnel: w746 -> [w753]
              tunnel: w745 -> [w750]
              tunnel: w744 -> [w749]
              tunnel: w743 -> [w748]
              tunnel: w742 -> [w752]
              frame #0 {
                n521 = global write "断电保存全局.vi" "IP"(w750) -> ()
                n522 = global write "断电保存全局.vi" "PORT"(w749) -> ()
                n523 = global write "断电保存全局.vi" "VISA Resource"(w751) -> ()
                n524 = global write "断电保存全局.vi" "MB通信方式选择"(w748) -> ()
                n525 = Enqueue Element(queue=w753, element=cluster{"命令":string} {"命令"="启用模块"} ("元素"), error in (no error)=w752) -> ()  [unwired: 1 in, 3 out]
              }
              frame #1 {
                n526 = call <vilib>:"Application Directory.vi"() -> ("Application Directory"=w768:path)
                n527 = Build Path(base path=w768, name or relative path="data\\sys.ini" ("名称或相对路径")) -> (appended path=w766:path)
                n528 = call <vilib>:"Open Config Data.vi"("configuration file path"=w766) -> ("error out"=w762:errorcluster, "refnum"=w765:T3)  [unwired: 8 in, 1 out]
                n529 = vi-ref "质控单元.lvlib:断电保存全局.vi"() -> (w764:refnum<vi>)
                n530 = call <userlib>:"Write Panel to INI__ogtk.vi"("error in (no error)"=w762, "VI ref"=w764, "refnum"=w765) -> ("error out"=w761:errorcluster, "refnum out"=w763:T3)  [unwired: 7 in]
                n531 = call <vilib>:"Close Config Data.vi"("error in (no error)"=w761, "refnum"=w763) -> ("error out"=w756:errorcluster, "file path"=w755:path)  [unwired: 8 in]
                n532 = Open/Create/Replace File(file path (use dialog)=w755, error in=w756) -> (refnum out=w759:refnum<file>, error out=w760:errorcluster)  [unwired: 4 in, 1 out]
                n533 = Flush File(refnum=w759, error in=w760) -> (refnum out=w758:refnum<file>, error out=w757:errorcluster)
                n534 = Close File(refnum=w758, error in=w757) -> ()  [unwired: 2 out]
              }
            }
          }
        }
      }
      event "释放串口": Value Change {
        n535 = event-data() -> ()  [unwired: 1 in, 6 out]
        n536 = Two Button Dialog(message="确认是否释放串口，释放串口将导致通信失败！" ("消息")) -> (T button?=w771:bool)  [unwired: 2 in]
        n537 = case shown="真" w771 {
          tunnel: w770 -> [_ w774]
          tunnel: w769 -> [_ w773]
          frame False {
          }
          frame True {
            n538 = Bundle By Name(cluster=cluster{"命令":string} {"命令"=""} ("元素"), "命令"="停用模块" ("名称（未命名）")) -> (w775:cluster{"命令":string})
            n539 = Enqueue Element(queue=w774, element=w775, error in (no error)=w773) -> ()  [unwired: 1 in, 3 out]
          }
        }
      }
      event "加标回收": Value Change {
        n540 = event-data() -> ()  [unwired: 1 in, 6 out]
        n541 = Send Notification(notification=FALSE ("通知"), notifier=w780) -> ()  [unwired: 1 in, 2 out]
        n542 = call "质控启动流程对话框.vi"() -> ("确定启动"=w778:bool, "启动模块"=w783:T8, "直接启动"=w781:bool, "常规启动"=w782:bool)  [unwired: 8 in]
        n543 = case shown="真" w778 {
          tunnel: w783 -> [_ w792]
          tunnel: w782 -> [_ w791]
          tunnel: w781 -> [_ w790]
          frame False {
          }
          frame True {
            n544 = Bundle By Name(cluster=T9 {"是否启用仪器"=FALSE, "CODMn"={"启动测量模式"={"测量模式"=enum."水样测量"}, "确定按钮"=FALSE}, "启动模块"={"氨氮"=FALSE, "总磷"=FALSE, "总氮"=FALSE, "CODMn"=FALSE, "CODCr"=FALSE}, "常规启动"=FALSE, "直接启动"=FALSE} ("参数"), "是否启用仪器"=TRUE, "启动模块"=w792, "常规启动"=w791, "直接启动"=w790) -> (w784:T9)
            n545 = vi-ref "质控单元.lvlib:一体站流程质控自动启动.vi"() -> (w787:refnum<vi>)
            n546 = property class="VI"(reference=w787) -> ("Name"=w788:string, "Exec.State"=w786:T12)  [unwired: 1 in, 2 out]
            n547 = case shown="\"Idle\"" w786 {
              tunnel: w788 -> [_ w803 _ _]
              tunnel: w784 -> [_ w793 _ _]
              frame "Bad", Default {
              }
              frame "Idle" {
                n548 = Open VI Reference(type specifier VI Refnum (for type only)=refnum<vi> refnum ("类型说明符VI引用句柄（仅用于类型）"), vi path=w803, options=128 ("选项")) -> (vi reference=w804:refnum<vi>, error out=w800:errorcluster)  [unwired: 3 in]
                n549 = call-by-ref "开始异步调用"(reference=w804, error in=w800, "CODMn量程切换"="CODMn量程选择", "总磷量程切换"="总磷量程选择", "总氮量程切换"="总氮量程选择", "氨氮量程切换"="氨氮量程选择", "参数"=w793) -> (reference out=w802:refnum<vi>, error out=w801:errorcluster)  [unwired: 7 in]
                n550 = Close Reference(reference=w802, error in (no error)=w801) -> ()  [unwired: 1 out]
              }
              frame "Run top level" {
              }
              frame "Running" {
                n551 = One Button Dialog(message="流程已启动，无需重复启动！" ("消息")) -> ()  [unwired: 1 in, 1 out]
              }
            }
          }
        }
      }
      event "报警清除": Value Change {
        w806 = u16 259 ("starting address")
        w812 = FALSE ("氨氮中断报警")
        n552 = event-data() -> ()  [unwired: 1 in, 6 out]
        n553 = global write "质控中断报警全局.vi" "氨氮中断报警"(w812) -> ()
        n554 = global write "质控中断报警全局.vi" "CODMn中断报警"(w812) -> ()
        n555 = global write "质控中断报警全局.vi" "总氮中断报警"(w812) -> ()
        n556 = global write "质控中断报警全局.vi" "总磷中断报警"(w812) -> ()
        n557 = global write "质控中断报警全局.vi" "CODCr中断报警"(w812) -> ()
        n558 = local read "氨氮模块"() -> (w816:bool)
        n559 = case shown="真" w816 {
          tunnel: [errorcluster {"status"=FALSE, "code"=0, "source"=""} ("error out") w841] -> w813
          tunnel: w806 -> [_ w840]
          frame False {
          }
          frame True {
            n560 = call "单个写入.vi"("value"=u16 0, "address"=w840, "Slave ID"=u8 1) -> ("error out"=w841:errorcluster)  [unwired: 8 in]
          }
        }
        n561 = local read "总磷模块选择"() -> (w815:bool)
        n562 = case shown="真" w815 {
          tunnel: w813 -> [w833 w836]
          tunnel: [w833 w835] -> w808
          tunnel: w806 -> [_ w834]
          frame False {
          }
          frame True {
            n563 = call "单个写入.vi"("Error in"=w836, "value"=u16 0, "address"=w834, "Slave ID"=u8 2) -> ("error out"=w835:errorcluster)  [unwired: 7 in]
          }
        }
        n564 = local read "总氮模块选择"() -> (w809:bool)
        n565 = case shown="真" w809 {
          tunnel: w808 -> [w817 w820]
          tunnel: [w817 w819] -> w807
          tunnel: w806 -> [_ w818]
          frame False {
          }
          frame True {
            n566 = call "单个写入.vi"("Error in"=w820, "value"=u16 0, "address"=w818, "Slave ID"=u8 3) -> ("error out"=w819:errorcluster)  [unwired: 7 in]
          }
        }
        n567 = local read "CODMn选择"() -> (w814:bool)
        n568 = case shown="真" w814 {
          tunnel: w807 -> [w827 w830]
          tunnel: [w827 w829] -> w810
          tunnel: w806 -> [_ w828]
          frame False {
          }
          frame True {
            n569 = call "单个写入.vi"("Error in"=w830, "value"=u16 0, "address"=w828, "Slave ID"=u8 4) -> ("error out"=w829:errorcluster)  [unwired: 7 in]
          }
        }
        n570 = local read "CODCr选择"() -> (w811:bool)
        n571 = case shown="真" w811 {
          tunnel: w810 -> [_ w824]
          tunnel: w806 -> [_ w823]
          frame False {
          }
          frame True {
            n572 = call "单个写入.vi"("Error in"=w824, "value"=u16 0, "address"=w823, "Slave ID"=u8 5) -> ()  [unwired: 7 in, 1 out]
          }
        }
      }
      event "平行样测试": Value Change {
        n573 = event-data() -> ()  [unwired: 1 in, 6 out]
        n574 = Cancel Notification(0:w847) -> ()  [unwired: 1 in, 3 out]
        n575 = call "平行样启动流程对话框.vi"() -> ("启动模块"=w846:T13, "常规启动"=w844:bool, "确定启动"=w845:bool)  [unwired: 9 in]
        n576 = case shown="真" w845 {
          tunnel: w846 -> [_ w854]
          tunnel: w844 -> [_ w849]
          frame False {
          }
          frame True {
            n577 = Bundle By Name(cluster=T10 {"参数启用"={"CODMn"=FALSE, "总磷"=FALSE, "总氮"=FALSE, "氨氮"=FALSE, "CODcr"=FALSE}, "采配水是否启动"=FALSE} ("参数"), "参数启用"=w854, "采配水是否启动"=w849) -> (w848:T10)
            n578 = vi-ref "质控单元.lvlib:一体站流程平行样自动启动.vi"() -> (w852:refnum<vi>)
            n579 = property class="VI"(reference=w852) -> ("Name"=w853:string, "Exec.State"=w851:T12)  [unwired: 1 in, 2 out]
            n580 = case shown="\"Idle\"" w851 {
              tunnel: w853 -> [_ w861]
              tunnel: w848 -> [_ w855]
              frame "Bad", Default {
              }
              frame "Idle" {
                n581 = Open VI Reference(type specifier VI Refnum (for type only)=refnum<vi> refnum ("类型说明符VI引用句柄（仅用于类型）"), vi path=w861, options=128 ("选项")) -> (vi reference=w862:refnum<vi>, error out=w860:errorcluster)  [unwired: 3 in]
                n582 = call-by-ref "开始异步调用"(reference=w862, error in=w860, "参数"=w855) -> (reference out=w857:refnum<vi>, error out=w856:errorcluster)  [unwired: 11 in]
                n583 = Close Reference(reference=w857, error in (no error)=w856) -> ()  [unwired: 1 out]
              }
            }
          }
        }
      }
      event "停止测量": Value Change {
        w865 = TRUE ("氨氮")
        # "停止采配水、氨氮、总磷总氮、COD、质控"
        n584 = event-data() -> ()  [unwired: 1 in, 6 out]
        n585 = call "质控启动参数选择对话框.vi"("CODCr"=w865, "CODMn"=w865, "总氮"=w865, "总磷"=w865, "氨氮"=w865) -> ("确定启动"=w866:bool, "启动模块"=w867:T8)  [unwired: 4 in, 1 out]
        n586 = case shown="真" w866 {
          tunnel: w867 -> [_ w877]
          tunnel: w864 -> [_ w870]
          tunnel: w863 -> [_ w868]
          frame False {
          }
          frame True {
            n587 = Send Notification(notification=TRUE ("通知"), notifier=w868) -> ()  [unwired: 1 in, 2 out]
            n588 = Unbundle By Name(w877) -> ("氨氮"=w875:bool, "总磷"=w873:bool, "总氮"=w872:bool, "CODMn"=w876:bool, "CODCr"=w874:bool)
            n589 = Enqueue Element At Opposite End(queue=w870, element=T11 {"命令"="单个写入", {"starting address"=300, "holding register value"=2}} ("元素")) -> ()  [unwired: 2 in, 3 out]
            n590 = case shown="假" w873 {
              frame False {
              }
              frame True {
                n591 = call "加标仪器启动命令 (子VI).vi"("启动命令"=enum16{"启动水样流程", "启动加标流程", "排液", "停止"}."停止", "仪器"=enum16{"", "氨氮", "总磷", "总氮", "CODMn", "CODCr"}."总磷") -> ()  [unwired: 9 in, 1 out]
                n592 = Obtain Queue(name (unnamed)="TP" ("名称（未命名）"), element data type=cluster{"命令":string, "data":variant} {"命令"="", "data"=variant}) -> (queue out=w903:refnum<queue>)  [unwired: 3 in, 2 out]
                n593 = Obtain Notifier(name (unnamed)="TP" ("名称（未命名）"), notification data type=FALSE) -> (notifier out=w899:refnum<notifier>)  [unwired: 2 in, 2 out]
                n594 = Send Notification(notification=TRUE ("通知"), notifier=w899) -> ()  [unwired: 1 in, 2 out]
                n595 = Enqueue Element(queue=w903, element=cluster{"命令":string, "data":variant} {"命令"="启动", "data"=variant(cluster{"站号":u16, "控制命令输出":u16[]} {"站号"=1, "控制命令输出"=[2816]})} ("元素")) -> ()  [unwired: 2 in, 3 out]
              }
            }
            n596 = case shown="真" w872 {
              frame False {
              }
              frame True {
                n597 = call "加标仪器启动命令 (子VI).vi"("启动命令"=enum16{"启动水样流程", "启动加标流程", "排液", "停止"}."停止", "仪器"=enum16{"", "氨氮", "总磷", "总氮", "CODMn", "CODCr"}."总氮") -> ()  [unwired: 9 in, 1 out]
                n598 = Obtain Queue(name (unnamed)="TN" ("名称（未命名）"), element data type=cluster{"命令":string, "data":variant} {"命令"="", "data"=variant}) -> (queue out=w887:refnum<queue>)  [unwired: 3 in, 2 out]
                n599 = Obtain Notifier(name (unnamed)="TN" ("名称（未命名）"), notification data type=FALSE) -> (notifier out=w883:refnum<notifier>)  [unwired: 2 in, 2 out]
                n600 = Send Notification(notification=TRUE ("通知"), notifier=w883) -> ()  [unwired: 1 in, 2 out]
                n601 = Enqueue Element(queue=w887, element=cluster{"命令":string, "data":variant} {"命令"="启动", "data"=variant(cluster{"站号":u16, "控制命令输出":u16[]} {"站号"=1, "控制命令输出"=[2816]})} ("元素")) -> ()  [unwired: 2 in, 3 out]
              }
            }
            n602 = case shown="真" w876 {
              frame False {
              }
              frame True {
                n603 = call "CODMn停止命令 (子VI).vi"() -> ()  [unwired: 12 in]
                n604 = Obtain Notifier(name (unnamed)="CODMn" ("名称（未命名）"), notification data type=FALSE) -> (notifier out=w916:refnum<notifier>)  [unwired: 2 in, 2 out]
                n605 = Send Notification(notification=TRUE ("通知"), notifier=w916) -> ()  [unwired: 1 in, 2 out]
                n606 = call "加标仪器启动命令 (子VI).vi"("启动命令"=enum16{"启动水样流程", "启动加标流程", "排液", "停止"}."停止", "仪器"=enum16{"", "氨氮", "总磷", "总氮", "CODMn", "CODCr"}."CODMn") -> ()  [unwired: 9 in, 1 out]
              }
            }
            n607 = case shown="真" w874 {
              frame False {
              }
              frame True {
                n608 = call "CODCr停止命令 (子VI).vi"() -> ()  [unwired: 12 in]
                n609 = Obtain Notifier(name (unnamed)="CODCr" ("名称（未命名）"), notification data type=FALSE) -> (notifier out=w890:refnum<notifier>)  [unwired: 2 in, 2 out]
                n610 = Send Notification(notification=TRUE ("通知"), notifier=w890) -> ()  [unwired: 1 in, 2 out]
                n611 = call "加标仪器启动命令 (子VI).vi"("启动命令"=enum16{"启动水样流程", "启动加标流程", "排液", "停止"}."停止", "仪器"=enum16{"", "氨氮", "总磷", "总氮", "CODMn", "CODCr"}."CODCr") -> ()  [unwired: 9 in, 1 out]
              }
            }
            n612 = case shown="真" w875 {
              frame False {
              }
              frame True {
                n613 = call "加标仪器启动命令 (子VI).vi"("启动命令"=enum16{"启动水样流程", "启动加标流程", "排液", "停止"}."停止", "仪器"=enum16{"", "氨氮", "总磷", "总氮", "CODMn", "CODCr"}."氨氮") -> ()  [unwired: 9 in, 1 out]
                n614 = Obtain Notifier(name (unnamed)="NH3N" ("名称（未命名）"), notification data type=FALSE) -> (notifier out=w909:refnum<notifier>)  [unwired: 2 in, 2 out]
                n615 = Obtain Queue(name (unnamed)="NH3N" ("名称（未命名）"), element data type=cluster{"命令":string, "data":variant} {"命令"="", "data"=variant}) -> (queue out=w913:refnum<queue>)  [unwired: 3 in, 2 out]
                n616 = Send Notification(notification=TRUE ("通知"), notifier=w909) -> ()  [unwired: 1 in, 2 out]
                n617 = Enqueue Element(queue=w913, element=cluster{"命令":string, "data":variant} {"命令"="启动", "data"=variant(cluster{"站号":u16, "控制命令输出":u16[]} {"站号"=1, "控制命令输出"=[2816]})} ("元素")) -> ()  [unwired: 2 in, 3 out]
              }
            }
          }
        }
      }
      event "定时启动": Value Change {
        n618 = event-data() -> ()  [unwired: 1 in, 6 out]
        n619 = flat-sequence {
          frame #0 {
            n620 = global read "断电保存全局.vi" "定时控制"() -> (w920:T6)
            n621 = call "周期设置.vi"("定时控制参数输入"=w920) -> ("定时控制参数输出"=w921:T6)  [unwired: 10 in]
            n622 = global write "断电保存全局.vi" "定时控制"(w921) -> ()
          }
          frame #1 {
            n623 = call <vilib>:"Application Directory.vi"() -> ("Application Directory"=w935:path)
            n624 = Build Path(base path=w935, name or relative path="data\\sys.ini" ("名称或相对路径")) -> (appended path=w933:path)
            n625 = call <vilib>:"Open Config Data.vi"("configuration file path"=w933) -> ("error out"=w929:errorcluster, "refnum"=w932:T3)  [unwired: 8 in, 1 out]
            n626 = vi-ref "质控单元.lvlib:断电保存全局.vi"() -> (w931:refnum<vi>)
            n627 = call <userlib>:"Write Panel to INI__ogtk.vi"("error in (no error)"=w929, "VI ref"=w931, "refnum"=w932) -> ("error out"=w928:errorcluster, "refnum out"=w930:T3)  [unwired: 7 in]
            n628 = call <vilib>:"Close Config Data.vi"("error in (no error)"=w928, "refnum"=w930) -> ("error out"=w923:errorcluster, "file path"=w922:path)  [unwired: 8 in]
            n629 = Open/Create/Replace File(file path (use dialog)=w922, error in=w923) -> (refnum out=w926:refnum<file>, error out=w927:errorcluster)  [unwired: 4 in, 1 out]
            n630 = Flush File(refnum=w926, error in=w927) -> (refnum out=w925:refnum<file>, error out=w924:errorcluster)
            n631 = Close File(refnum=w925, error in=w924) -> ()  [unwired: 2 out]
          }
        }
      }
      event "查看": Value Change {
        n632 = event-data() -> ()  [unwired: 1 in, 6 out]
        n633 = property on="窗格" class="Pane"("Origin"=T2 {"Horizontal"=0, "Vertical"=640} ("原点")) -> ()  [unwired: 2 in, 2 out]
      }
      event "返回": Value Change {
        n634 = event-data() -> ()  [unwired: 1 in, 6 out]
        n635 = property on="窗格" class="Pane"("Origin"=T2 {"Horizontal"=0, "Vertical"=0} ("原点")) -> ()  [unwired: 2 in, 2 out]
      }
    }
  }
  n636 = call-by-ref "?"(reference=w34, error in=w36) -> (reference out=w38:refnum<vi>, error out=w37:errorcluster)  [unwired: 12 in]
  n637 = Open VI Reference(type specifier VI Refnum (for type only)=refnum<vi> refnum, vi path=w25, options=128 ("选项")) -> (vi reference=w23:refnum<vi>, error out=w21:errorcluster)  [unwired: 3 in]
  n638 = call-by-ref "?"(reference=w23, error in=w21) -> (reference out=w19:refnum<vi>, error out=w20:errorcluster)  [unwired: 12 in]
  n639 = Close Reference(reference=w38, error in (no error)=w37) -> ()  [unwired: 1 out]
  n640 = call-by-ref "?"(reference=w15, error in=w13, "CODMn"=w7, "总磷"=w8, "CODCr"=w6, "氨氮"=w9, "总氮"=w10) -> (reference out=w11:refnum<vi>, error out=w12:errorcluster)  [unwired: 7 in]
  n641 = Close Reference(reference=w19, error in (no error)=w20) -> ()  [unwired: 1 out]
  n642 = Close Reference(reference=w11, error in (no error)=w12) -> ()  [unwired: 1 out]
